vi "DataAcqMaster.vi"(0 "Motion Settings In":T4={"No Motion?"=FALSE, "Motion System"=enum."NI 735x", "Motion Bd ID"=1, "Motion Profile"="SMAC1", "# Axis"=1, "Reverse Z axis?"=TRUE, "SMAC Axis"=0, "scan pair"=enum."y-(x) scan", "RT fps"=6.0, "Steps per mm"=[1000, 1000, 1000, 1000], "Motor Parameters"={"velocity ct/s"=[10000.0, 10000.0, 10000.0, 50000.0], "accel ct/s^2"=[50000.0, 50000.0, 50000.0, 200000.0]}, "One Way Scan"=FALSE, "Reverse One Way Scan"=FALSE, "Global Position (mm)"=[], "Plane"=0, "Distance between\nscan lines (um)"=0.0, "Distance between\nscan planes (um)"=0.0, "number of scan planes"=1, "Total steps in line"=0, "Xtra plane\ndistance  (um)"=100, "Xtra planes "=1, "Add Axis"=FALSE, "overshoot cts"=200, "BKPT Shift"=0, "Scan Start Time (ms)"=0, "ESP VISA"="GPIB::1::INSTR", "3rd Axis"=1, "GL Ref Out"=refnum, "Galil Address"=""} {"3rd Axis" items=["x", "y", "z", "w"]; "Xtra planes" min=1; "Xtra plane\ndistance  (um)" min=0; "Distance between\nscan planes (um)" format="%.2f"; "Distance between\nscan lines (um)" format="%.2f"; "SMAC Axis" items=["None"=0, "Axis 1"=1, "Axis 2"=2, "Axis 3"=3, "Axis 4"=4, "Axis 5"=5, "Axis 6"=6, "Axis 7"=7, "Axis 8"=8, "Vector Space 1"=17, "Vector Space 2"=18, "Vector Space 3"=19, "Vector Space 4"=20]; "Motion Bd ID" min=1 max=32 step=1}, 1 "2-D motor":bool, 2 "Type of scan":T12, 3 "Move motor":bool, 5 "Therapy (T)":bool, 6 "Scan Name":string, 7 "Xmit Ring":i16, 8 "Digitizer Settings":T8={"Digitizer delay (us) "=0.0, "rf points per line"=2048, "lines per plane"=128, "Samp Rate (Hz)"=100000000.0, "Additional dig delay (us)"=0.0, "Voltage Scale"=0.4, "Pre-Looks"=0, "Offset delay (us)"=0.0, "bits A/D"=8, "Avg Num"=1, "DigTimeOut"=5.0, "Rel Dig Delay"=0.0, "Dig Ch"=0, "LeCroyCluster"={"LeCroy Channels"=[TRUE, FALSE, FALSE, FALSE], "LC read pt offset"=0.0, "Sweep Avg"=FALSE}, "Main Digitizer"=enum."NI Digitizer", "Dig Config"=enum."Single channel", "Digitizer ID Cluster"={"Acqiris/Alazar/SP ID"=[], "NI Instr Handles"=[], "LeCroy VISA"="", "GaGe Handle"={"Handle"=0, "Sample size"=0, "Resolution"=0, "Offset"=0, "Channels"=0, "Boards"=0}, "ATS Ref"="ATS9350", "Acqiris Address"=["PCI::INSTR0"], "ADQRef"=refnum, "adq_cu_ptr"=refnum}, "Trigger Settings"={"Trig Source"=1, "Trig Coupling"=0, "Trig Slope"=0, "Level (mV)"=1500.0}, "Bulk Acq"=FALSE, "Bulk Start Indexes"=[], "Data Ref RF"=refnum, "NI ID/Channel"=[], "Total Dig CH"=1, "Xtra Ann Trig delay (us)"=10.0, "Fix Z Delay?"=FALSE, "One Way Transmission?"=FALSE, "Data Ref Log"=refnum} {"Trigger Settings"."Trig Slope" items=["Positive", "Negative"]; "Trigger Settings"."Level (mV)" format="%.2f"; "Trigger Settings"."Trig Coupling" items=["DC 1 MOhm", "AC 1 MOhm", "DC 50 Ohm", "AC 50 Ohm"]; "Trigger Settings"."Trig Source" items=["Chan 1", "External"]; "Rel Dig Delay" format="%.2f"; "DigTimeOut" format="%.2f"; "Avg Num" min=1; "Offset delay (us)" format="%.2f"; "Additional dig delay (us)" format="%.2f"; "Digitizer delay (us)" format="%.2f"}, 10 "lines per plane mod":i32, 12 "Ann Array Params":T1={"Synth Foc?"=FALSE, "Focal Zones"=41, "Switch T/R"=0, "Trans Geometry (mm)"={"Transducer"=0, "Geo Focus"=12.0, "a (radius)"=3.0, "# of rings"=5, "kerf space "=0.1, "Center Freq"=12.0}, "Sub Ap Excite?"=FALSE, "Full Array Scan?"=FALSE, "Xmt/Rcv"={"XMIT"=[TRUE, TRUE, TRUE, TRUE, TRUE], "RCV"=[TRUE, TRUE, TRUE, TRUE, TRUE]}, "PulseSpacing (us)"=0.0, "Xmit Ring"=0, "XMIT CHS"=0, "RCV CHS"=0, "GPU?"=FALSE, "Save TIFF?"=FALSE, "downfactor"=1, "RCV 1CH"=0} {"RCV 1CH" items=["All", "1", "2", "3", "4", "5"]; "Trans Geometry (mm)"."Transducer" items=["6D 12R 40 MHz"=0, "10D 31R 20 MHz"=1, "10D 23R 20 MHz"=2, "6D 23R 40 MHz"=3, "4.5D 10.7R 40 MHz"=4, "9D 23.5R 20 MHz"=5, "9D 25.8R 20MHz"=6, "Enter"=99]; "Switch T/R" min=1 max=5 step=1}, 13 "Reverse ?":bool, 14 "DAQmx Task 2":refnum<k21>, 15 "Full Array Scan?":bool, 16 "start value":dbl, 18 "scan axis":i32) -> (17 "Stop Scan":bool, 21 "Motion error":bool, 22 "Timeout":bool, 26 "error out":errorcluster, 27 "Record Index":i32)   [LabVIEW 2022 SP3]
uses:
  Controls/ScanType2.ctl
  Digitizers/-DigitizerRoutines/DigitizerSettings.ctl
  Digitizers/-DigitizerRoutines/Digitizer.ctl
  Digitizers/-DigitizerRoutines/DigConfig.ctl
  Digitizers/-DigitizerRoutines/DigitizerID.ctl
  C:/Windows/System32/ADQAPI_dotNet_helper.dll
  Windows/System32/ADQAPI_dotNet_helper.dll
  Motion Controllers/NI_controller/-NI_MotionRoutines/MotionParameters.ctl
  Motion Controllers/NI_controller/-NI_MotionRoutines/MotionSys.ctl
  Motion Controllers/-MotionRoutines/ScanAxis.ctl
  Motion Controllers/-MotionRoutines/3rdAxis.ctl
  Annular Array/-AnnularRoutines/AnnularArray.ctl
  Annular Array/-AnnularRoutines/TransGeometry.ctl
  Annular Array/-AnnularRoutines/ArrayGeometry.ctl
  Motion Controllers/Galil/Command Menu.ctl
  Controls/location.ctl
  <vilib>/DAQmx/write.llb/DAQmx Write (Digital Bool 1Line 1Point).vi
  <vilib>/DAQmx/read.llb/DAQmx Read (Analog 2D I16 NChan NSamp).vi
  Motion Controllers/-MotionRoutines/MotionGlobals.vi
  Pulsers/PulserGlobals.vi
  <vilib>/DAQmx/miscellaneous.llb/DAQmx Fill In Error Info.vi
  Switch Modules/SwitchGlobals.vi
  <instrlib>/Acqiris Dx/Acqiris Dx.lvlib
  <vilib>/Motion/FlexMotion/FunctionsVIs/Trajectory.llb/Wait for Move Complete (8 axes).flx
  <resource>/objmgr/daqmx.rc
  <vilib>/Motion/FlexMotion/CustomControls/CustomControls.llb/Mask (8 axes).flx
  <instrlib>/Newport ESP301/Newport ESP301.lvlib
  <instrlib>/LeCroy Wave Series/LeCroy Wave Series.lvlib
  <instrlib>/Agilent 34970/Agilent 34970.lvlib
  <vilib>/Motion/FlexMotion/FunctionsVIs/MotionIO.llb/Set Breakpoint Output MOMO (8 axes).flx
  <vilib>/Motion/FlexMotion/FunctionsVIs/MotionIO.llb/Set Inhibit MOMO (8 axes).flx
panel:
  out "TEMP Log 2":bool
  # "1-D and 2-D B scan settings"
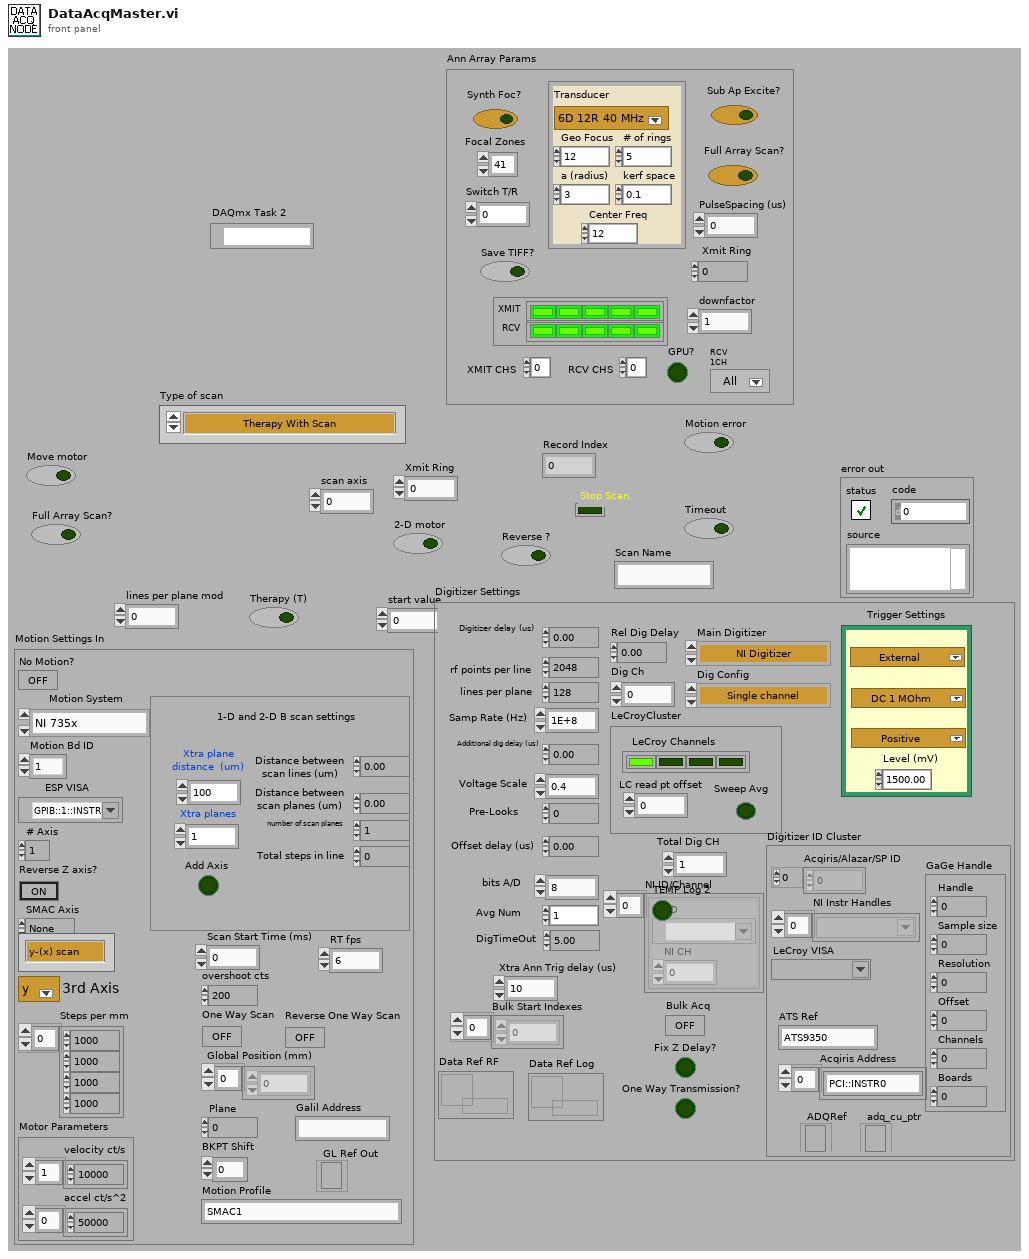
[diagram p1: front panel]
types:
  T1 = typedef "AnnularArray.ctl" = cluster{"Synth Foc?":bool, "Focal Zones":i16, "Switch T/R":i16, "Trans Geometry (mm)":T2, "Sub Ap Excite?":bool, "Full Array Scan?":bool, "Xmt/Rcv":cluster{"XMIT":bool[], "RCV":bool[]}, "PulseSpacing (us)":sgl, "Xmit Ring":i32, "XMIT CHS":u8, "RCV CHS":u8, "GPU?":bool, "Save TIFF?":bool, "downfactor":i32, "RCV 1CH":u16}
  T2 = typedef "TransGeometry.ctl" = cluster{"Transducer":T3, "Geo Focus":dbl, "a (radius)":dbl, "# of rings":i32, "kerf space ":dbl, "Center Freq":dbl}
  T3 = typedef "ArrayGeometry.ctl" = u16
  T4 = typedef "MotionParameters.ctl" = cluster{"No Motion?":bool, "Motion System":T5, "Motion Bd ID":u8, "Motion Profile":string, "# Axis":i8, "Reverse Z axis?":bool, "SMAC Axis":u16, "scan pair":T6, "RT fps":sgl, "Steps per mm":i32[], "Motor Parameters":cluster{"velocity ct/s":dbl[], "accel ct/s^2":dbl[]}, "One Way Scan":bool, "Reverse One Way Scan":bool, "Global Position (mm)":dbl[], "Plane":i32, "Distance between\nscan lines (um)":sgl, "Distance between\nscan planes (um)":sgl, "number of scan planes":i32, "Total steps in line":i32, "Xtra plane\ndistance  (um)":i32, "Xtra planes ":i32, "Add Axis":bool, "overshoot cts":i32, "BKPT Shift":i32, "Scan Start Time (ms)":u32, "ESP VISA":refnum<visa-resource-name>, "3rd Axis":T7, "GL Ref Out":refnum<k7>, "Galil Address":string}
  T5 = typedef "MotionSys.ctl" = enum16{"MM3000", "NI 735x", "Newport ESP", "No Motion Card", "Galil"}
  T6 = typedef "ScanAxis.ctl" = enum16{"y-(x) scan", "x-(y) scan", "z-(x) scan", "z-(y) scan", "y-(z) scan", "x-(z) scan", "w-(x) scan", "w-(y) scan", "w-(z) scan", "x-(w) scan", "y-(w) scan", "z-(w) scan"}
  T7 = typedef "3rdAxis.ctl" = u16
  T8 = typedef "DigitizerSettings.ctl" = cluster{"Digitizer delay (us) ":dbl, "rf points per line":i32, "lines per plane":i32, "Samp Rate (Hz)":dbl, "Additional dig delay (us)":dbl, "Voltage Scale":dbl, "Pre-Looks":i32, "Offset delay (us)":dbl, "bits A/D":i8, "Avg Num":i32, "DigTimeOut":sgl, "Rel Dig Delay":sgl, "Dig Ch":i32, "LeCroyCluster":cluster{"LeCroy Channels":bool[], "LC read pt offset":dbl, "Sweep Avg":bool}, "Main Digitizer":T9, "Dig Config":T10, "Digitizer ID Cluster":T11, "Trigger Settings":cluster{"Trig Source":u16, "Trig Coupling":u16, "Trig Slope":u16, "Level (mV)":dbl}, "Bulk Acq":bool, "Bulk Start Indexes":i32[], "Data Ref RF":refnum<data-value>, "NI ID/Channel":cluster{"NI ID":refnum<k15>, "NI CH":i32}[], "Total Dig CH":i32, "Xtra Ann Trig delay (us)":dbl, "Fix Z Delay?":bool, "One Way Transmission?":bool, "Data Ref Log":refnum<data-value>}
  T9 = typedef "Digitizer.ctl" = enum16{"Acqiris Digitizer", "NI Digitizer", "LeCroy", "GaGe", "AlazarTech", "No Digitizer", "Teledyne"}
  T10 = typedef "DigConfig.ctl" = enum16{"Single channel", "2 Chans w/ 2 Acqiris", "2 Chans w/ 1 Acqiris", "5-CH Pulser New", "5-CH pulser w/ ann array", "5-pass style ann array", "Empty"}
  T11 = typedef "DigitizerID.ctl" = cluster{"Acqiris/Alazar/SP ID":u32[], "NI Instr Handles":refnum<k15>[], "LeCroy VISA":refnum<visa-resource-name>, "GaGe Handle":cluster{"Handle":u32, "Sample size":u32, "Resolution":i32, "Offset":i32, "Channels":u32, "Boards":u32}, "ATS Ref":string, "Acqiris Address":string[], "ADQRef":refnum<k24>, "adq_cu_ptr":refnum<k24>}
  T12 = typedef "ScanType2.ctl" = enum16{"Therapy With Scan", "M scan", "M Scan With Therapy Burst", "1-D B Scan", "1-D B Scan With Therapy Burst", "2-D B Scan", "2-D B Scan With Therapy Burst", "Rotational Scan", "1-D B-Scan PRF", "2-D B-Scan PRF", "Real-Time Scan", "Contrast Agents", "1-D w/ Real-Time Set Up", "Dual Transducer", "Acoustic Microscopy", "Hydrophone Scanning"}
  T13 = typedef "EKG_Mode.ctl" = u16
  T14 = typedef "Mask (8 axes).flx" = cluster{"1":bool, "2":bool, "3":bool, "4":bool, "5":bool, "6":bool, "7":bool, "8":bool}
  T15 = typedef "Command Menu.ctl" = enum16{"CommandPassThrough", "Abort Motion", "Define Pos", "Velocity", "Acceleration", "Deceleration", "Position Rel", "Postion Abs", "Begin Move", "After Move", "Home", "KI", "KD", "KP", "IL", "Config I/O", "Set Bit", "Clear Bit", "Motor Off", "Moto On", "Status", "Execute", "Halt Execute", "HX Status", "Tell Velocity", "Check Motion", "BreakPoint", "Tell Position", "Current Code Line", "Tell Switches", "OC Force On", "OC Off", "Pos Soft Limit", "Rev Soft Limit"}
  T16 = typedef "location.ctl" = enum16{"Automatic", "WCM Main", "Hawaii", "Columbia MM3000", "Columbia  NI System", "NYU", "RRI 2", "UHI Allen", "CUMC RT", "Chiba", "Stony Brook", "WCM Microscopy", "WCM Aeoretch", "WCM Optics Lab", "WCM Main 2Axis", "WCM Rotation", "WCM SAM SMAC", "SERI GP"}
  T17 = cluster{dbl, "Clock mode":enum16{"Internal", "External", "Reference"}, "RingText.Text":string, i32, i32, "time out (ms)":dbl, dbl, dbl}
  T18 = enum16{"big-endian, network order", "native, host order", "little-endian"}
  T19 = enum16{"open", "replace", "create", "open or create", "replace or create", "replace or create with confirmation"}
  T20 = cluster{"Therapy frequency (MHz)":dbl, "Therapy amplitude (mV)":dbl, "time therapy on (s)":dbl, "Therapy Delay (ms) ":dbl, "Time (s)":dbl}
  T21 = enum32{"unused", "DC, 1 MOhm", "AC, 1 MOhm", "DC, 50 Ohm", "AC 50 Ohm"}
  T22 = cluster{"Handle":u32, "Sample size":u32, "Resolution":i32, "Offset":i32, "Channels":u32, "Boards":u32}
  T23 = cluster{"Voltage Scale":dbl, "Voltage Scale":dbl, "Crate Coupling":u16}
  T24 = cluster{"data value reference":refnum<data-value>, "bytes to transfer":u32, "rf pts actual":u32}
  T25 = cluster{"Port A bit-0 at logic level":bool, "Port A bit-1 at logic level":bool, "Port A bit-2 at logic level ":bool, "Port A bit-3 at logic level":bool, "Port A bit-4 at logic level":bool, "Port A bit-5 at logic level ":bool, "Port A bit-6 at logic level ":bool, "Port A bit-7 at logic level ":bool, "Port B bit-0 at logic level":bool, "Port B bit-1 at logic level":bool, "Port B bit-2 at logic level ":bool, "Port B bit-3 at logic level":bool, "Port B bit-4 at logic level":bool, "Port B bit-5 at logic level ":bool, "Port B bit-6 at logic level ":bool, "Port B bit-7 at logic level ":bool}
  T26 = typedef "SwitchOption.ctl" = enum16{"Cytex", "Pickering", "NI Switch", "No Switch", "Riverside USB"}
  T27 = typedef "Bd Id Out" = u8
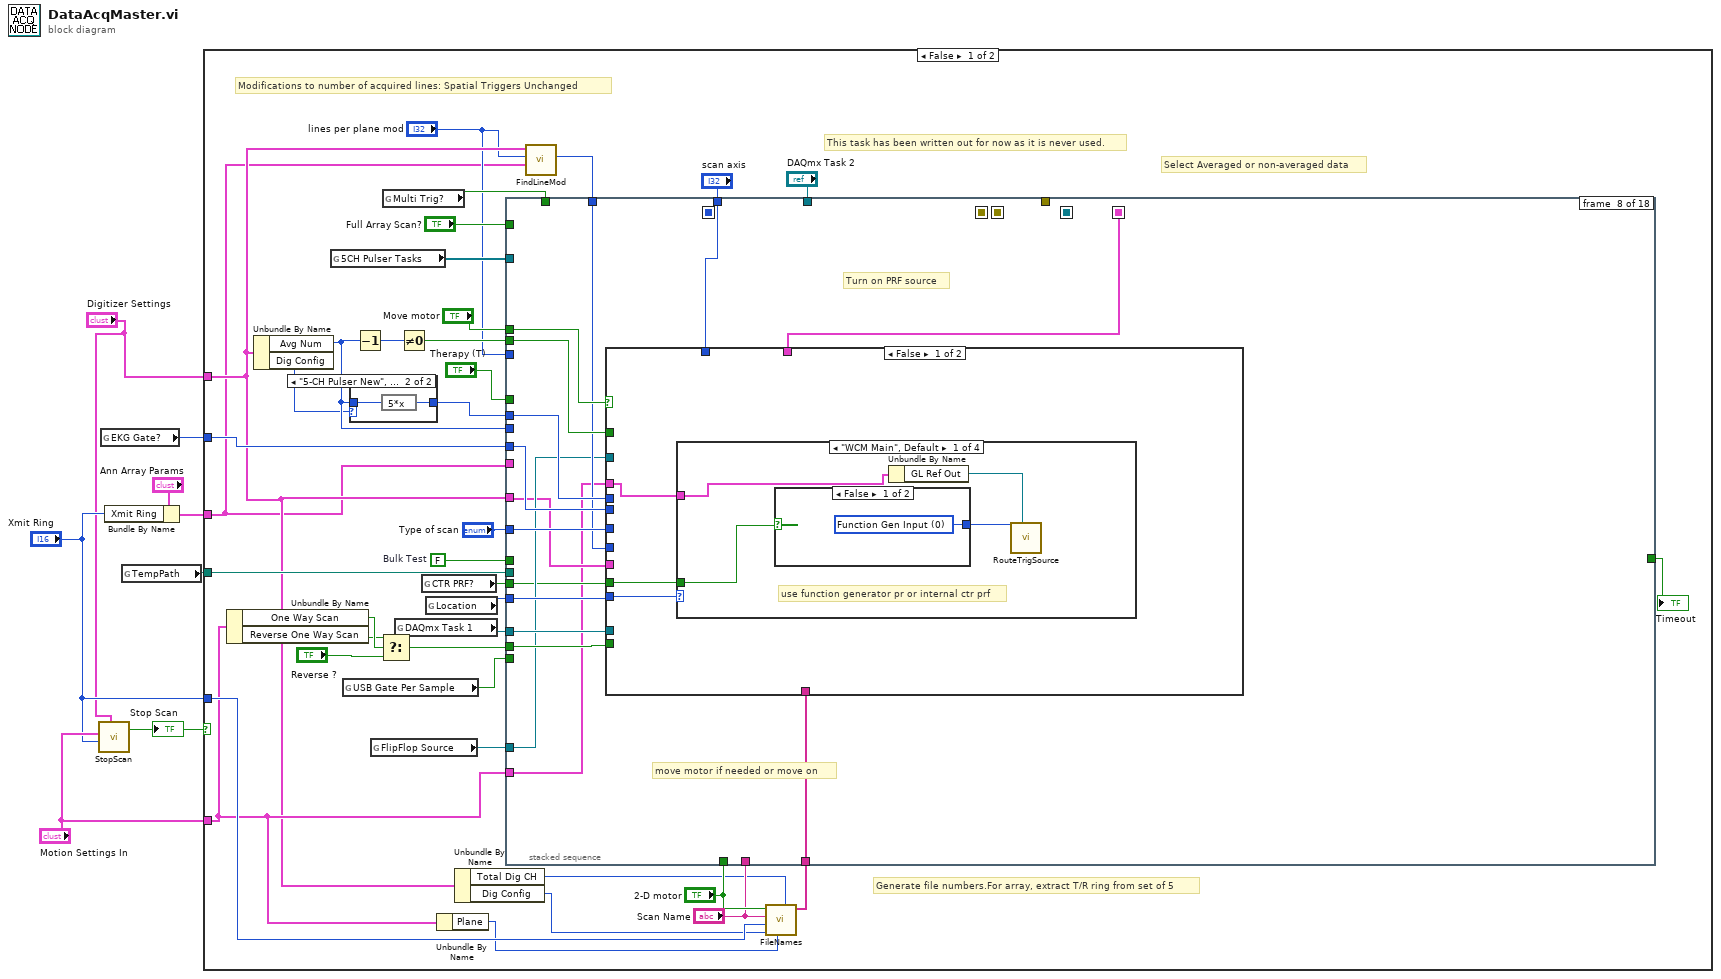
[diagram p0: block diagram]
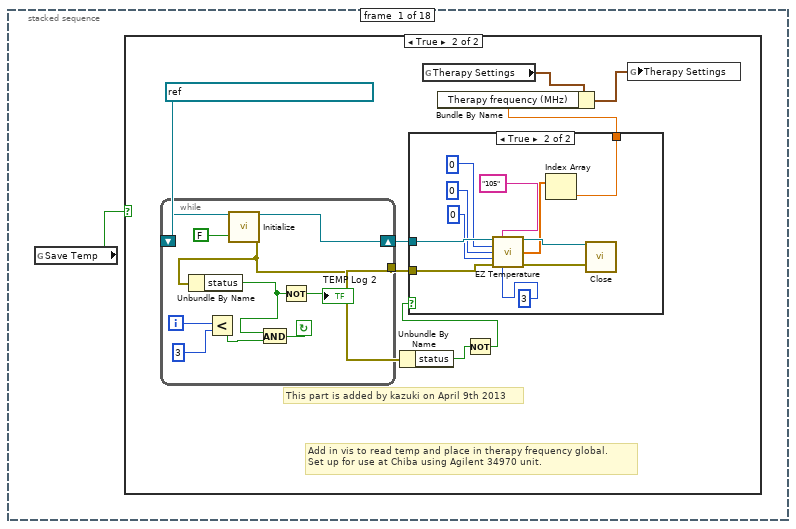
[diagram p3: hidden frame]
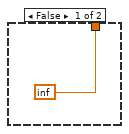
[diagram p5: hidden frame]
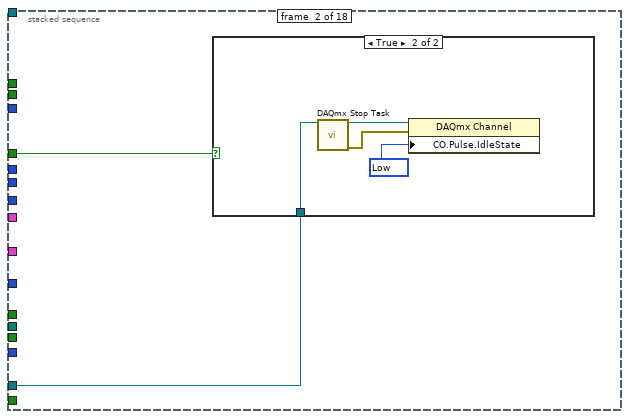
[diagram p6: hidden frame]
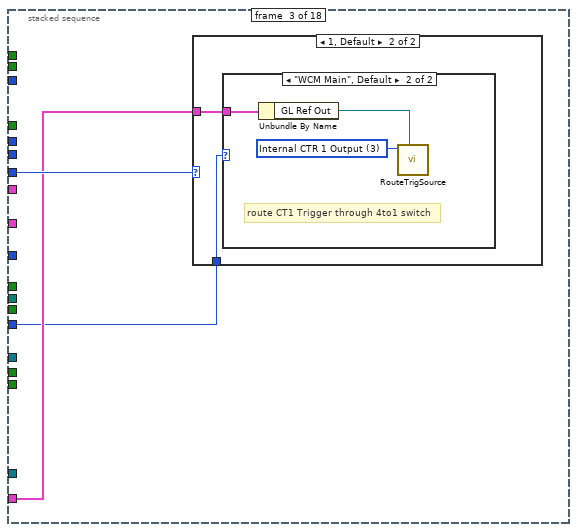
[diagram p8: hidden frame]
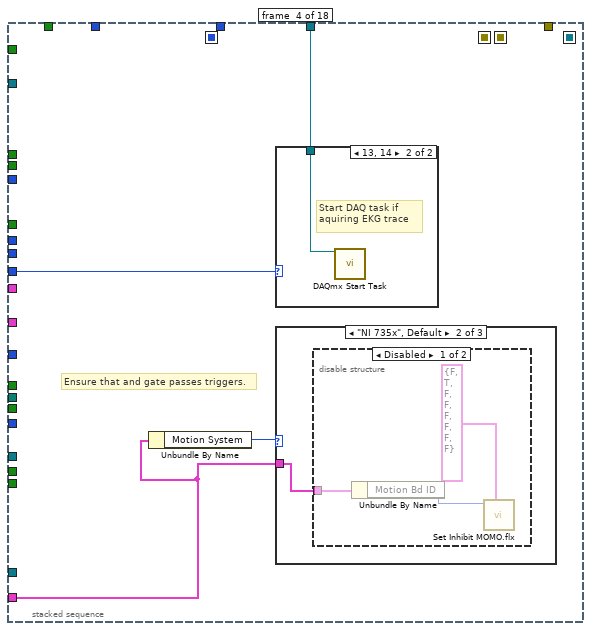
[diagram p11: hidden frame]
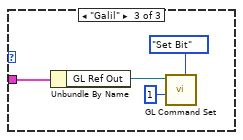
[diagram p14: hidden frame]
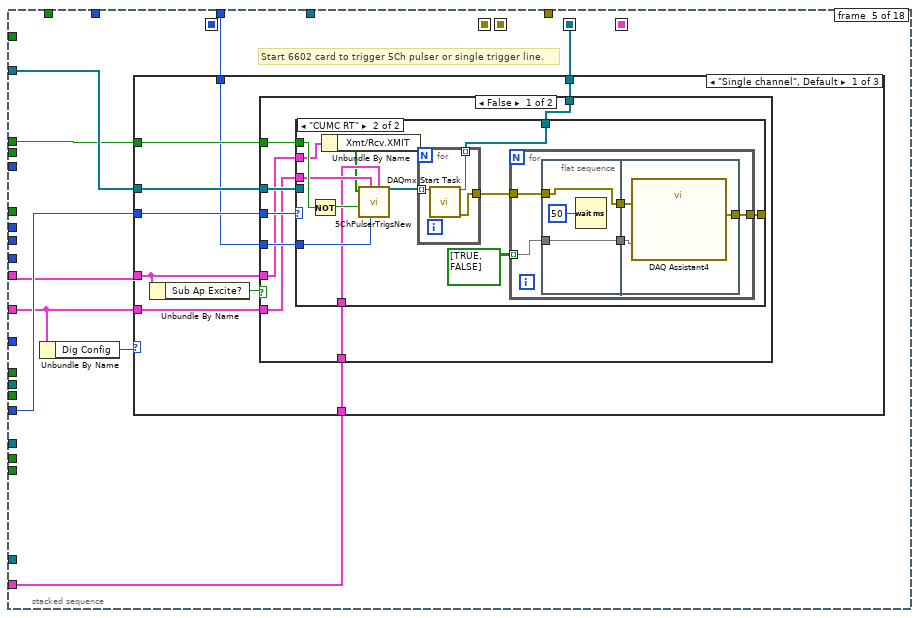
[diagram p16: hidden frame]
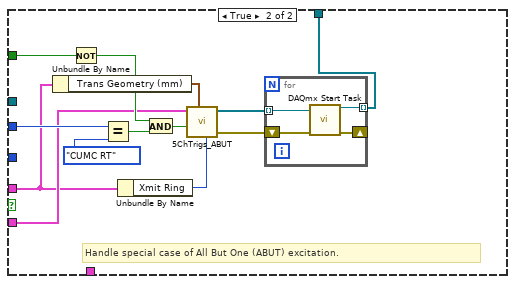
[diagram p18: hidden frame]
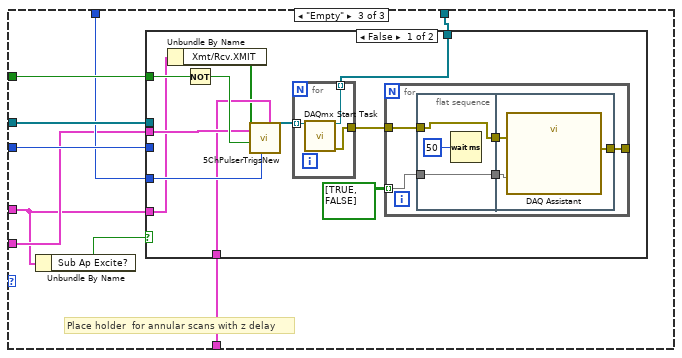
[diagram p20: hidden frame]
diagram:
  n1 = call "StopScan.vi"("Motion Settings In"="Motion Settings In", "Ring"="Xmit Ring", "Digitizer Settings"="Digitizer Settings") -> ("Stop Now? Dup"=w8:bool)  [unwired: 3 in]
  "Stop Scan" <- w8
  n2 = global read "MotionGlobals.vi" "EKG Gate?"() -> (w7:T13)
  n3 = Bundle By Name(cluster="Ann Array Params", "Xmit Ring"="Xmit Ring") -> (w2:T1)
  n4 = global read "MotionGlobals.vi" "TempPath"() -> (w6:path)
  n5 = case shown="False" w8 {
    tunnel: "Xmit Ring" -> [w16 _]
    tunnel: w7 -> [w46 _]
    tunnel: w6 -> [w28 _]
    tunnel: "Digitizer Settings" -> [w11 _]
    tunnel: "Motion Settings In" -> [w14 _]
    tunnel: w2 -> [w9 _]
    frame False {
      w32 = FALSE  # Bulk Test
      # "This task has been written out for now as it is never used."
      # "Modifications to number of acquired lines: Spatial Triggers Unchanged"
      # "Generate file numbers.For array, extract T/R ring from set of 5"
      # "Select Averaged or non-averaged data"
      n6 = Unbundle By Name(w14) -> ("One Way Scan"=w20:bool, "Reverse One Way Scan"=w18:bool)
      n7 = Unbundle By Name(w11) -> ("Avg Num"=w22:i32, "Dig Config"=w21:T10)
      n8 = global read "MotionGlobals.vi" "5CH Pulser Tasks"() -> (w29:refnum<k21>[])
      n9 = global read "MotionGlobals.vi" "USB Gate Per Sample"() -> (w19:bool)
      n10 = case shown="\"5-CH Pulser New\", \"5-CH pulser w/ ann array\"" w21 {
        tunnel: [w47 w49] -> w27
        tunnel: w22 -> [w47 w48]
        frame "Single channel", Default {
        }
        frame "5-CH Pulser New", "5-CH pulser w/ ann array" {
          n11 = expression code="5*x"(w48) -> (w49:i32)
        }
      }
      n12 = Decrement(x=w22) -> (x-1=w40:i32)
      n13 = global read "MotionGlobals.vi" "FlipFlop Source"() -> (w26:refnum<k21>)
      n14 = Select(t=w18, s=w20, f="Reverse ?") -> (s? t:f=w35:bool)
      n15 = global read "MotionGlobals.vi" "Multi Trig?"() -> (w23:bool)
      n16 = global read "MotionGlobals.vi" "DAQmx Task 1"() -> (w37:refnum<k21>)
      n17 = Not Equal To 0?(x=w40) -> (x != 0?=w41:bool)
      n18 = global read "MotionGlobals.vi" "CTR PRF?"() -> (w25:bool)
      n19 = global read "MotionGlobals.vi" "Location"() -> (w39:T16)
      n20 = Unbundle By Name(w14) -> ("Plane"=w13:i32)
      n21 = Unbundle By Name(w11) -> ("Total Dig CH"=w17:i32, "Dig Config"=w15:T10)
      n22 = call "FindLineMod.vi"("Ann Array Params"=w9, "lines per plane in"="lines per plane mod", "Digitizer Settings"=w11) -> ("lines per plane mod out"=w24:i32)  [unwired: 8 in]
      n23 = call "FileNames.vi"("# Elements"=w17, "Plane"=w13, "Dig Config"=w15, "Xmit Ring"=w16, "Scan Name"="Scan Name", "2-D motor"="2-D motor") -> ("All files"=w34:string[])  [unwired: 3 in, 2 out]
      n24 = stacked-sequence {
        seq-local: [_ _ _ _ _ w245 _ _ _ _ _ _ _ _ _ _ _ _] -> [_ _ _ _ _ _ _ _ w566 _ _ _ _ _ _ _ _ _]
        seq-local: [_ _ _ _ _ _ _ _ w559 _ _ _ _ _ _ _ _ _] -> [_ _ _ _ _ _ _ _ _ w635 w682 _ _ _ _ _ _ _]
        seq-local: [_ _ _ _ _ w241 _ _ _ _ _ _ _ _ _ _ _ _] -> [_ _ _ _ _ _ _ _ w563 w633 w680 _ _ _ _ _ _ _]
        seq-local: [_ _ _ _ w113 _ _ _ _ _ _ _ _ _ _ _ _ _] -> [_ _ _ _ _ _ _ _ _ _ _ _ _ w803 _ _ _ _]
        seq-local: [_ _ _ _ _ w236 _ _ _ _ _ _ _ _ _ _ _ _] -> [_ _ _ _ _ _ _ w464 _ _ w674 _ _ _ _ _ _ w1004]
        tunnel: "Therapy (T)" -> [_ w81 _ _ _ _ w453 _ _ _ _ _ w779 _ _ _ _ _]
        tunnel: "Move motor" -> [_ _ _ _ w114 _ w450 w477 _ _ _ _ w776 _ _ w872 _ _]
        tunnel: "scan axis" -> [_ _ _ _ w112 _ _ w475 _ _ w677 _ _ _ _ w868 w931 _]
        tunnel: w35 -> [_ _ _ _ _ _ _ w476 _ w634 w681 _ _ _ _ w870 _ _]
        tunnel: [_ _ _ _ _ _ _ _ w565 _ _ _ _ _ _ _ _ _] -> w45
        tunnel: "Type of scan" -> [_ _ _ _ _ _ w447 w472 _ w625 w670 _ w774 _ _ _ w926 _]
        tunnel: w41 -> [_ _ _ _ _ w243 _ w474 _ _ _ _ _ _ _ _ _ _]
        tunnel: w27 -> [_ _ _ _ _ w244 _ w473 w564 _ _ _ _ _ _ _ _ _]
        tunnel: w39 -> [_ _ w87 _ w115 _ w444 w471 _ _ _ _ w770 w804 _ w871 _ _]
        tunnel: w37 -> [_ w82 _ _ _ _ w455 w467 _ _ _ _ w783 _ _ _ _ _]
        tunnel: w46 -> [_ _ w89 w98 _ _ _ w470 _ w632 w679 _ w782 _ w825 w869 w928 _]
        tunnel: w24 -> [_ _ _ _ _ w242 _ w469 w562 _ _ _ _ _ _ _ _ _]
        tunnel: w23 -> [_ _ _ _ _ _ w454 _ _ _ _ _ w771 _ _ _ _ _]
        tunnel: w34 -> [_ _ _ _ _ _ _ w468 _ _ w678 _ _ _ w824 _ _ _]
        tunnel: "Full Array Scan?" -> [_ _ _ _ _ _ _ _ _ _ _ w754 _ _ _ _ _ _]
        tunnel: "DAQmx Task 2" -> [_ _ _ w97 _ _ _ _ _ _ _ _ _ _ w823 _ _ _]
        tunnel: w32 -> [_ _ _ _ _ _ _ _ _ w631 w676 _ _ _ _ _ _ _]
        tunnel: "2-D motor" -> [_ _ _ _ _ _ _ _ _ w630 _ _ _ _ _ _ _ _]
        tunnel: "Scan Name" -> [_ _ _ _ _ _ _ _ _ w629 _ _ _ _ _ _ _ _]
        tunnel: w29 -> [_ _ _ _ w116 _ _ _ _ _ _ _ _ _ _ _ _ _]
        tunnel: w28 -> [_ _ _ _ _ _ _ _ _ _ _ _ _ _ w822 _ _ _]
        tunnel: w22 -> [_ _ _ _ _ w237 _ _ _ _ w675 _ _ _ _ _ _ _]
        tunnel: w26 -> [_ _ _ _ _ _ _ w466 _ _ _ _ _ _ _ _ _ w1005]
        tunnel: w25 -> [_ _ _ _ _ _ w451 w465 _ _ _ _ w778 _ _ _ _ _]
        tunnel: w11 -> [_ _ _ _ w109 w230 _ w463 w561 w628 w673 w750 _ w801 w821 _ _ w1000]
        tunnel: w14 -> [_ _ w88 w96 w111 w231 _ w462 _ w627 w672 _ w772 _ _ w867 w924 w1003]
        tunnel: w19 -> [_ _ _ _ _ _ w448 _ w560 _ _ _ _ _ _ _ _ _]
        tunnel: w9 -> [_ _ _ _ w110 w235 _ _ _ w626 w671 w752 _ w802 w820 _ _ _]
        tunnel: [_ _ _ _ _ _ _ _ w559 _ _ _ _ _ _ _ _ _] -> _
        tunnel: "lines per plane mod" -> [_ _ _ _ _ _ _ _ _ _ _ _ _ _ w819 _ _ _]
        frame #0 {
          n25 = global read "MotionGlobals.vi" "Save Temp"() -> (w50:bool)
          n26 = case shown="True" w50 {
            frame False {
            }
            frame True {
              # "This part is added by kazuki on April 9th 2013"
              # "Add in vis to read temp and place in therapy frequency global.\nSet up for use at Chiba using Agilent 34970 unit."
              n27 = while {
                tunnel: [w77] -> w56
                shift-right: [w79] -> w58
                shift-left: refnum<visa-resource-name> "TCPIP0::192.168.1.170::inst0::INSTR" ("VISA Resource Name") -> [w78]
                i -> [w74]
                stop <- w76 continue-if-true
                n28 = Less?(x=w74, y=3) -> (x < y?=w75:bool)
                n29 = call <instrlib>:"Initialize.vi"("VISA Resource Name"=w78, "Reset (T: Reset)"=FALSE) -> ("VISA Resource Name Out"=w79:refnum<visa-resource-name>, "error out"=w77:errorcluster)  [unwired: 12 in]
                n30 = Unbundle By Name(w77) -> ("status"=w71:bool)
                n31 = And(x=w71, y=w75) -> (x .and. y?=w76:bool)
                n32 = Not(x=w71) -> (.not. x?=→"TEMP Log 2":bool)
              }
              n33 = Unbundle By Name(w56) -> ("status"=w55:bool)
              n34 = global read "PulserGlobals.vi" "Therapy Settings"() -> (w53:T20)
              n35 = Not(x=w55) -> (.not. x?=w54:bool)
              n36 = case shown="True" w54 {
                tunnel: [inf w67] -> w52
                tunnel: w58 -> [_ w65]
                tunnel: w56 -> [_ w60]
                frame False {
                }
                frame True {
                  n37 = call <instrlib>:"EZ Temperature.vi"("VISA Resource Name"=w65, "Scan List (empty)"="105", "Thermocouple Type (8:Def-Last)"=0, "Thermistor Type (3:Def-Last)"=0, "RTD Type (2:Default-Last)"=0, "error in (no error)"=w60, "Transducer Type (4:Def-Last)"=3) -> ("VISA Resource Name Out"=w69:refnum<visa-resource-name>, "Output Array"=w68:dbl[], "error out"=w70:errorcluster)  [unwired: 6 in]
                  n38 = Index Array(array=w68) -> (element=w67:dbl)  [unwired: 1 in]
                  n39 = call <instrlib>:"Close.vi"("VISA Resource Name"=w69, "error in (no error)"=w70) -> ()  [unwired: 13 in, 1 out]
                }
              }
              n40 = Bundle By Name(cluster=w53, "Therapy frequency (MHz)"=w52) -> (w51:T20)
              n41 = global write "PulserGlobals.vi" "Therapy Settings"(w51) -> ()
            }
          }
        }
        frame #1 {
          n42 = case shown="True" w81 {
            tunnel: w82 -> [_ w86]
            frame False {
            }
            frame True {
              w83 = 10214 items=["High"=10192, "Low"=10214] ("CO.Pulse.IdleState")
              n43 = call <vilib>:"DAQmx Stop Task.vi"("task/channels in"=w86) -> ("task out"=w85:refnum<k21>, "error out"=w84:errorcluster)  [unwired: 1 in, 12 out]
              n44 = property class="DAQmx Channel"(reference=w85, error in=w84, "CO.Pulse.IdleState"=w83) -> ()  [unwired: 2 out]
            }
          }
        }
        frame #2 {
          n45 = case shown="1, Default" w89 {
            tunnel: w88 -> [_ w91]
            tunnel: w87 -> [_ w90]
            frame 0 {
            }
            frame 1, Default {
              n46 = case shown="\"WCM Main\", Default" w90 {
                tunnel: w91 -> [_ w93]
                frame "SERI GP" {
                }
                frame "WCM Main", Default {
                  w94 = u16 3 items=["Function Gen Input", "Motion Trig", "Internal RT Motion Trig", "Internal CTR 1 Output"] ("Trig Source")
                  # "route CT1 Trigger through 4to1 switch"
                  n47 = Unbundle By Name(w93) -> ("GL Ref Out"=w92:refnum<k7>)
                  n48 = call "RouteTrigSource.vi"("Galil.IGalil"=w92, "Trig Source"=w94) -> ()  [unwired: 9 in, 1 out]
                }
              }
            }
          }
        }
        frame #3 {
          # "Ensure that and gate passes triggers."
          n49 = Unbundle By Name(w96) -> ("Motion System"=w95:T5)
          n50 = case shown="13, 14" w98 {
            tunnel: w97 -> [_ w107]
            frame 0, Default {
            }
            frame 13, 14 {
              # "Start DAQ task if aquiring EKG trace"
              n51 = call <vilib>:"DAQmx Start Task.vi"("task/channels in"=w107) -> ()  [unwired: 1 in, 14 out]
            }
          }
          n52 = case shown="\"NI 735x\", Default" w95 {
            tunnel: w96 -> [_ w99 w104]
            frame "MM3000", "Newport ESP", "No Motion Card" {
            }
            frame "NI 735x", Default {
              n53 = disable-structure shown="Disabled" {
                disable-tunnel: w99 -> [w101 _]
                frame Disabled {
                  n54 = Unbundle By Name(w101) -> ("Motion Bd ID"=w100:u8)
                  n55 = call-poly <vilib>:"Set Inhibit MOMO.flx"("Must On (False)"=T14 {"1"=FALSE, "2"=TRUE, "3"=FALSE, "4"=FALSE, "5"=FALSE, "6"=FALSE, "7"=FALSE, "8"=FALSE}, "Board ID"=w100) -> ()  [unwired: 2 in, 6 out]
                }
                frame Enabled {
                }
              }
            }
            frame "Galil" {
              n56 = Unbundle By Name(w104) -> ("GL Ref Out"=w106:refnum<k7>)
              n57 = call "GL Command Set.vi"("Command"=Command_Menu."Set Bit", "Value"=1, "Galil.IGalil"=w106) -> ()  [unwired: 4 in, 5 out]
            }
          }
        }
        frame #4 {
          # "Start 6602 card to trigger 5Ch pulser or single trigger line."
          n58 = Unbundle By Name(w109) -> ("Dig Config"=w108:T10)
          n59 = case shown="\"Single channel\", Default" w108 {
            tunnel: w116 -> [w124 w177 w185]
            tunnel: w115 -> [w125 _ w186]
            tunnel: w114 -> [w123 _ w184]
            tunnel: [w122 w177 w183] -> w113
            tunnel: w112 -> [w121 _ w182]
            tunnel: w109 -> [w118 _ w181]
            tunnel: w111 -> [w120 _ w180]
            tunnel: w110 -> [w117 _ w178]
            frame "Single channel", Default {
              n60 = Unbundle By Name(w117) -> ("Sub Ap Excite?"=w119:bool)
              n61 = case shown="False" w119 {
                tunnel: w125 -> [w133 w168]
                tunnel: w124 -> [w132 _]
                tunnel: w123 -> [w130 w171]
                tunnel: [w129 w165] -> w122
                tunnel: w121 -> [w131 _]
                tunnel: w118 -> [w128 w164]
                tunnel: w120 -> [w127 _]
                tunnel: w117 -> [w126 w160]
                frame False {
                  n62 = case shown="\"CUMC RT\"" w133 {
                    tunnel: w132 -> [_ _]
                    tunnel: w131 -> [_ w144]
                    tunnel: w130 -> [_ w143]
                    tunnel: [_ w141] -> w129
                    tunnel: [_ w138] -> _
                    tunnel: w128 -> [_ w137]
                    tunnel: w127 -> [_ w136]
                    tunnel: w126 -> [_ w134]
                    frame "WCM Main", Default {
                    }
                    frame "CUMC RT" {
                      n63 = Not(x=w143) -> (.not. x?=w145:bool)
                      n64 = Unbundle By Name(w134) -> ("Xmt/Rcv.XMIT"=w135:bool[])
                      n65 = call "5ChPulserTrigsNew.vi"("Motion Settings"=w136, "Digitizer Settings"=w137, "XMIT"=w135, "Axis"=w144, "M-mode?"=w145) -> ("5CH Pulser Tasks"=w142:refnum<k21>[])  [unwired: 4 in, 1 out]
                      n66 = for {
                        tunnel: w142 -> [w159] mode=indexing
                        tunnel: [w158] -> w141 mode=indexing
                        tunnel: [w157] -> w139
                        n67 = call <vilib>:"DAQmx Start Task.vi"("task/channels in"=w159) -> ("task out"=w158:refnum<k21>, "error out"=w157:errorcluster)  [unwired: 1 in, 12 out]
                      }
                      n68 = for {
                        tunnel: bool[][] [[TRUE], [FALSE]] ("data") -> [w149] mode=indexing
                        tunnel: [w148] -> w138
                        tunnel: w139 -> [w146]
                        n69 = flat-sequence {
                          tunnel: w149 -> [w153]
                          tunnel: [w153] -> w150
                          tunnel: [w151] -> w147
                          tunnel: w146 -> [w151]
                          tunnel: w150 -> [w156]
                          tunnel: [w155] -> w148
                          tunnel: w147 -> [w154]
                          frame #0 {
                            n70 = Wait (ms)(milliseconds to wait=u32 50) -> ()  [unwired: 1 out]
                          }
                          frame #1 {
                            n71 = call "DAQ Assistant4"("data"=w156, "error in"=w154) -> ("error out"=w155:errorcluster)  [unwired: 16 in, 1 out]
                          }
                        }
                      }
                    }
                  }
                }
                frame True {
                  # "Handle special case of All But One (ABUT) excitation."
                  n72 = Unbundle By Name(w160) -> ("Trans Geometry (mm)"=w162:T2)
                  n73 = Not(x=w171) -> (.not. x?=w170:bool)
                  n74 = Equal?(x=w168, y=location."CUMC RT" ("Location")) -> (x = y?=w169:bool)
                  n75 = Unbundle By Name(w160) -> ("Xmit Ring"=w161:i32)
                  n76 = And(x=w170, y=w169) -> (x .and. y?=w167:bool)
                  n77 = call "5ChTrigs_ABUT.vi"("xmit ring"=w161, "Trans Geometry (mm)"=w162, "Digitizer Settings"=w164, "M-mode?"=w167) -> ("5CH Pulser Tasks"=w166:refnum<k21>[], "error out"=w172:errorcluster)  [unwired: 5 in]
                  n78 = for {
                    tunnel: w166 -> [w176] mode=indexing
                    shift-right: [w174] -> _
                    shift-left: w172 -> [w175]
                    tunnel: [w173] -> w165 mode=indexing
                    n79 = call <vilib>:"DAQmx Start Task.vi"("task/channels in"=w176, "error in"=w175) -> ("task out"=w173:refnum<k21>, "error out"=w174:errorcluster)  [unwired: 12 in]
                  }
                }
              }
            }
            frame "5-CH pulser w/ ann array" {
            }
            frame "Empty" {
              # "Place holder  for annular scans with z delay"
              n80 = Unbundle By Name(w178) -> ("Sub Ap Excite?"=w179:bool)
              n81 = case shown="False" w179 {
                tunnel: w186 -> [_ w220]
                tunnel: w185 -> [_ _]
                tunnel: w184 -> [w196 w223]
                tunnel: [w195 w217] -> w183
                tunnel: w182 -> [w197 _]
                tunnel: w181 -> [w190 w216]
                tunnel: w180 -> [w189 _]
                tunnel: w178 -> [w187 w212]
                frame False {
                  n82 = Unbundle By Name(w187) -> ("Xmt/Rcv.XMIT"=w188:bool[])
                  n83 = Not(x=w196) -> (.not. x?=w194:bool)
                  n84 = call "5ChPulserTrigsNew.vi"("Motion Settings"=w189, "Digitizer Settings"=w190, "XMIT"=w188, "Axis"=w197, "M-mode?"=w194) -> ("5CH Pulser Tasks"=w193:refnum<k21>[])  [unwired: 4 in, 1 out]
                  n85 = for {
                    tunnel: w193 -> [w211] mode=indexing
                    tunnel: [w210] -> w195 mode=indexing
                    tunnel: [w209] -> w191
                    n86 = call <vilib>:"DAQmx Start Task.vi"("task/channels in"=w211) -> ("task out"=w210:refnum<k21>, "error out"=w209:errorcluster)  [unwired: 1 in, 12 out]
                  }
                  n87 = for {
                    tunnel: bool[][] [[TRUE], [FALSE]] ("data") -> [w201] mode=indexing
                    tunnel: [w200] -> _
                    tunnel: w191 -> [w198]
                    n88 = flat-sequence {
                      tunnel: w201 -> [w205]
                      tunnel: [w205] -> w202
                      tunnel: [w203] -> w199
                      tunnel: w198 -> [w203]
                      tunnel: w202 -> [w208]
                      tunnel: [w207] -> w200
                      tunnel: w199 -> [w206]
                      frame #0 {
                        n89 = Wait (ms)(milliseconds to wait=u32 50) -> ()  [unwired: 1 out]
                      }
                      frame #1 {
                        n90 = call "DAQ Assistant"("data"=w208, "error in"=w206) -> ("error out"=w207:errorcluster)  [unwired: 16 in, 1 out]
                      }
                    }
                  }
                }
                frame True {
                  # "Handle special case of All But One (ABUT) excitation."
                  n91 = Not(x=w223) -> (.not. x?=w222:bool)
                  n92 = Unbundle By Name(w212) -> ("Xmit Ring"=w213:i32)
                  n93 = Equal?(x=w220, y=location."CUMC RT" ("Location")) -> (x = y?=w221:bool)
                  n94 = Unbundle By Name(w212) -> ("Trans Geometry (mm)"=w214:T2)
                  n95 = And(x=w222, y=w221) -> (x .and. y?=w219:bool)
                  n96 = call "5ChTrigs_ABUT.vi"("xmit ring"=w213, "Trans Geometry (mm)"=w214, "Digitizer Settings"=w216, "M-mode?"=w219) -> ("5CH Pulser Tasks"=w218:refnum<k21>[], "error out"=w224:errorcluster)  [unwired: 5 in]
                  n97 = for {
                    tunnel: w218 -> [w228] mode=indexing
                    shift-right: [w226] -> _
                    shift-left: w224 -> [w227]
                    tunnel: [w225] -> w217 mode=indexing
                    n98 = call <vilib>:"DAQmx Start Task.vi"("task/channels in"=w228, "error in"=w227) -> ("task out"=w225:refnum<k21>, "error out"=w226:errorcluster)  [unwired: 12 in]
                  }
                }
              }
            }
          }
        }
        frame #5 {
          n99 = Absolute Value(x=w244) -> (abs(x)=w238:i32)
          n100 = Unbundle By Name(w230) -> ("Bulk Acq"=w229:bool)
          n101 = Unbundle By Name(w235) -> ("Xmit Ring"=w234:i32)
          n102 = Unbundle By Name(w230) -> ("Main Digitizer"=w233:T9, "Dig Config"=w232:T10)
          n103 = Not Equal To 0?(x=w234) -> (x != 0?=w239:bool)
          n104 = Not And(1:w239, 2:w229) -> (0:w240:bool)
          n105 = Select(t=w238, s=w243, f=w242) -> (s? t:f=w241:i32)
          n106 = case shown="True" w240 {
            tunnel: [_ w255] -> w245
            tunnel: w232 -> [_ w248]
            tunnel: w243 -> [_ w253]
            tunnel: w241 -> [_ w254]
            tunnel: w237 -> [_ w251]
            tunnel: [_ w250] -> w236
            tunnel: w230 -> [_ w249]
            tunnel: w233 -> [_ w247]
            tunnel: w231 -> [_ w246]
            frame False {
            }
            frame True {
              # "set up A/D card for sequence acquistion using parameters selected earlier"
              n107 = case shown="\"2 Chans w/ 2 Acqiris\", Default" w248 {
                tunnel: w254 -> [_ w427]
                tunnel: [_ w428] -> w252
                tunnel: w253 -> [_ w426]
                tunnel: w247 -> [_ w425]
                tunnel: w249 -> [_ w424]
                frame "Single channel", "2 Chans w/ 1 Acqiris" {
                }
                frame "2 Chans w/ 2 Acqiris", Default {
                  n108 = Unbundle By Name(w424) -> ("rf points per line"=w423:i32)
                  n109 = case shown="\"Acqiris Digitizer\", Default" w425 {
                    tunnel: [w433 w443 _] -> w428
                    tunnel: w423 -> [w432 w441 _]
                    tunnel: w427 -> [w431 w442 _]
                    tunnel: w426 -> [w430 w440 _]
                    tunnel: w424 -> [w429 w439 _]
                    frame "Acqiris Digitizer", Default {
                      n110 = disable-structure shown="Disabled" {
                        disable-tunnel: [w438 _] -> w433
                        disable-tunnel: w432 -> [w437 _]
                        disable-tunnel: w431 -> [w436 _]
                        disable-tunnel: w430 -> [w435 _]
                        disable-tunnel: w429 -> [w434 _]
                        frame Disabled {
                          n111 = call "ArmCratePrams.vi"("Arm trig Not?"=w435, "num lines"=w436, "rf pts"=w437, "Digitizer Settings"=w434) -> ("error out"=w438:errorcluster)  [unwired: 10 in, 1 out]
                        }
                        frame Enabled {
                        }
                      }
                    }
                    frame "NI Digitizer" {
                      n112 = call "NIArmCratePrams.vi"("Arm Trig Not?"=w440, "num lines"=w442, "rf pts"=w441, "Digitizer Settings"=w439) -> ("error out"=w443:errorcluster)  [unwired: 11 in]
                    }
                    frame "LeCroy", "AlazarTech" {
                    }
                  }
                }
              }
              n113 = case shown="\"Acqiris Digitizer\"" w247 {
                tunnel: [w261 w297 w314 _ _ _ _] -> w255
                tunnel: w252 -> [w260 w289 _ _ _ _ _]
                tunnel: w253 -> [w259 w301 w333 w360 w384 w401 _]
                tunnel: w254 -> [w258 w303 w330 w361 w381 w396 _]
                tunnel: w251 -> [_ _ w317 _ _ _ _]
                tunnel: [_ _ _ _ _ w397 _] -> w250
                tunnel: w248 -> [_ _ _ _ _ w402 _]
                tunnel: w249 -> [w256 w291 w312 w343 w370 w391 _]
                tunnel: w246 -> [_ _ w309 _ _ _ _]
                frame "Acqiris Digitizer" {
                  n114 = Unbundle By Name(w256) -> ("Digitizer ID Cluster.Acqiris/Alazar/SP ID"=w257:u32[])
                  n115 = disable-structure shown="Disabled" {
                    disable-tunnel: [w282 _] -> w261
                    disable-tunnel: w260 -> [w281 _]
                    disable-tunnel: w259 -> [w280 _]
                    disable-tunnel: w258 -> [w279 _]
                    disable-tunnel: w257 -> [w278 _]
                    disable-tunnel: w256 -> [w273 _]
                    frame Disabled {
                      # "arm trigger"
                      # "set up for sequence"
                      n116 = Unbundle By Name(w273) -> ("rf points per line"=w262:i32, "Voltage Scale"=w272:dbl)
                      n117 = Index Array(array=w278) -> (element=w270:u32)  [unwired: 1 in]
                      n118 = call <instrlib>:"Query Vertical Settings.vi"("Instrument ID"=w270, "Channel (1)"=1) -> ("dup Instrument ID"=w268:u32, "Coupling"=w266:T21, "error out"=w269:errorcluster, "Offset"=w271:dbl)  [unwired: 2 in, 2 out]
                      n119 = To Word Integer(number=w266) -> (16bit integer=w264:i16)
                      n120 = Decrement(x=w264) -> (x-1=w265:i16)
                      n121 = call <instrlib>:"Configure Memory Settings.vi"("error in (no error)"=w269, "Number of Samples (1000)"=w262, "Number of Segments (1)"=w279, "Instrument ID"=w268) -> ("error out"=w275:errorcluster, "dup Instrument ID"=w277:u32)  [unwired: 2 out]
                      n122 = Bundle("Voltage Scale"=w272, "Offset"=w271, w265) -> (w267:cluster{"Voltage Scale":dbl, "Offset":dbl, i16})  [unwired: 1 in]
                      n123 = call "conVert.vi"("InstrumentID"=w277, "V scale"=w267, "error in"=w275) -> ("Status"=w276:i32, "error out"=w274:errorcluster)  [unwired: 2 in, 1 out]
                      n124 = call "conSamp.vi"("error in"=w274, "Digitizer Settings"=w273, "InstrumentID"=w276) -> ("error out"=w283:errorcluster, "DUP ID"=w284:u32)  [unwired: 1 in]
                      n125 = case shown="False" w280 {
                        tunnel: w284 -> [w287 _]
                        tunnel: w283 -> [w286 w288]
                        tunnel: [w285 w288] -> w282
                        tunnel: w281 -> [_ _]
                        frame False {
                          n126 = call <instrlib>:"Start Acquisition.vi"("error in (no error)"=w286, "Instrument ID"=w287) -> ("error out"=w285:errorcluster)  [unwired: 2 in, 1 out]
                        }
                        frame True {
                        }
                      }
                    }
                    frame Enabled {
                    }
                  }
                }
                frame "NI Digitizer", Default {
                  n127 = Unbundle By Name(w291) -> ("Digitizer ID Cluster.NI Instr Handles"=w294:refnum<k15>[])
                  n128 = Unbundle By Name(w291) -> ("rf points per line"=w290:i32)
                  n129 = Unbundle By Name(w291) -> ("Voltage Scale"=w293:dbl)
                  n130 = Index Array(array=w294) -> (element=w295:refnum<k15>)  [unwired: 1 in]
                  n131 = property class="niScope"(reference=w295, "Reference Position"=0, "Min Number of Points"=w290, "Number of Records"=w303, "Enable Records > Memory"=TRUE, "Vertical Range"=w293) -> (reference out=w300:refnum<k15>, error out=w292:errorcluster)  [unwired: 1 in]
                  n132 = call "NI conSamp.vi"("error in"=w292, "Digitizer Settings"=w291, "InstrumentID"=w300) -> ("error out"=w298:errorcluster, "DUP ID"=w299:refnum<k15>)  [unwired: 1 in]
                  n133 = case shown="False" w301 {
                    tunnel: w299 -> [w306 _]
                    tunnel: w298 -> [w305 w307]
                    tunnel: [w304 w307] -> w297
                    tunnel: w289 -> [_ _]
                    frame False {
                      n134 = call <instrlib>:"niScope Initiate Acquisition.vi"("instrument handle"=w306, "error in"=w305) -> ("error out"=w304:errorcluster)  [unwired: 1 in, 12 out]
                    }
                    frame True {
                    }
                  }
                }
                frame "LeCroy" {
                  w320 = u16 0 items=["RealTime", "RIS", "Sequence", "Roll", "WaveStream"] ("Sample Mode (0: RealTime)")
                  w329 = FALSE ("Continuous Acquisition Mode (T: On)")
                  w319 = u16 2 items=["RealTime", "RIS", "Sequence", "Roll", "WaveStream"] ("Sample Mode (0: RealTime)")
                  # "Need delay first time due to lag in LeCroy"
                  n135 = Unbundle By Name(w312) -> ("Digitizer delay (us)"=w313:dbl)
                  n136 = Unbundle By Name(w312) -> ("Digitizer ID Cluster.LeCroy VISA"=w311:refnum<visa-resource-name>)
                  n137 = call <instrlib>:"Configure Continuous Acquisition.vi"("Auto Trigger Enabled (T: Normal)"=w329, "Continuous Acquisition Mode (T: On)"=w329, "VISA resource name"=w311) -> ("error out"=w331:errorcluster, "VISA resource name out"=w332:refnum<visa-resource-name>)  [unwired: 7 in]
                  n138 = Equal?(x=-1 ("y"), y=w317) -> (x = y?=w310:bool)
                  n139 = expression code="-1E-6*x"(w313) -> (w327:dbl)
                  n140 = Select(t=w320, s=w310, f=w319) -> (s? t:f=w318:u16)
                  n141 = Number To Exponential String(number=w327) -> (E-format string=w328:string)  [unwired: 3 in]
                  n142 = call <instrlib>:"Configure Sample Mode.vi"("error in (no error)"=w331, "Number of Segments (2)"=w330, "Sample Mode (0: RealTime)"=w318, "VISA resource name"=w332) -> ("error out"=w325:errorcluster, "VISA resource name out"=w326:refnum<visa-resource-name>)  [unwired: 6 in]
                  n143 = Concatenate Strings("TRDL " ("Write Buffer"), w328) -> (w324:string)
                  n144 = call <instrlib>:"Write.vi"("error in (no error)"=w325, "Write Buffer"=w324, "VISA resource name"=w326) -> ("error out"=w322:errorcluster, "VISA resource name out"=w321:refnum<visa-resource-name>)  [unwired: 6 in, 1 out]
                  n145 = case shown="False" w333 {
                    tunnel: w321 -> [w339 _]
                    tunnel: w322 -> [w338 w340]
                    tunnel: [w337 w340] -> w315
                    frame False {
                      n146 = call <instrlib>:"Initiate.vi"("error in (no error)"=w338, "VISA resource name"=w339) -> ("error out"=w337:errorcluster)  [unwired: 8 in, 1 out]
                    }
                    frame True {
                    }
                  }
                  n147 = Unbundle By Name(w309) -> ("Plane"=w308:i32)
                  n148 = case shown="0" w308 {
                    tunnel: w315 -> [w334 w336]
                    tunnel: [w334 w336] -> w314
                    frame 0 {
                      n149 = Wait (ms)(milliseconds to wait=500) -> ()  [unwired: 1 out]
                    }
                    frame 1, Default {
                    }
                  }
                }
                frame "GaGe" {
                  w356 = 128
                  # "might need to update samp rate in but should occur only if predefined samp freqs are wrong"
                  # "USB version with no delay support. Must take too many pts"
                  n150 = Unbundle By Name(w343) -> ("rf points per line"=w341:i32, "Samp Rate (Hz)"=w345:dbl, "Digitizer delay (us)"=w346:dbl, "Additional dig delay (us)"=w347:dbl, "Offset delay (us)"=w348:dbl)
                  n151 = Unbundle By Name(w343) -> ("Digitizer ID Cluster.GaGe Handle"=w342:T22)
                  n152 = Compound Arithmetic op=ADD(w346, w347, w348) -> (w344:dbl)
                  n153 = Multiply(x=w345, y=w344) -> (x*y=w352:dbl)
                  n154 = expression code="x*1E-6"(w352) -> (w351:dbl)
                  n155 = Add(x=w341, y=w351) -> (x+y=w354:dbl)
                  n156 = Quotient & Remainder(x=w354, y=w356) -> (floor(x/y)=w355:dbl)  [unwired: 1 out]
                  n157 = Increment(x=w355) -> (x+1=w357:dbl)
                  n158 = Multiply(x=w357, y=w356) -> (x*y=w353:dbl)
                  n159 = Bundle(cluster=T17 {0.0, "Clock mode"=enum."Internal", "RingText.Text"="Single", 0, 0, "time out (ms)"=0.0, 0.0, 0.0} ("output cluster"), w345, w353, w353) -> (w362:T17)  [unwired: 5 in]
                  n160 = call "CsTool-ConfigureAcquisitionAll.vi"("Handle Cluster"=w342, "Segment Count (1)"=w361, "Acquisition"=w362) -> ("Error Code"=w358:i32)  [unwired: 2 in]
                  n161 = flat-sequence {
                    tunnel: [w365] -> w359
                    tunnel: w342 -> [w365]
                    tunnel: [w366] -> _
                    tunnel: w358 -> [_]
                    tunnel: [w365] -> w350
                    frame #0 {
                      w367 = TRUE
                      n162 = call "CsTool-CommitAll.vi"("OnlyOnChange (t)"=w367, "Coerce Flag (f)"=w367, "Handle Cluster"=w365) -> ("Error Code"=w366:i32)  [unwired: 1 out]
                    }
                  }
                  n163 = call "CsTool-QueryAcquisitionParametersFill.vi"("Handle Cluster"=w350) -> ("Sample Rate"=w349:dbl)  [unwired: 10 out]
                  n164 = case shown="False" w360 {
                    tunnel: w359 -> [w364 _]
                    frame False {
                      n165 = call "CsTool-CaptureFill.vi"("Handle Cluster"=w364) -> ()  [unwired: 1 out]
                    }
                    frame True {
                    }
                  }
                  n166 = Bundle By Name(cluster=w343, "Samp Rate (Hz)"=w349) -> ()  [unwired: 1 out]
                }
                frame "Teledyne" {
                  # "extra shift needed to hit delay"
                  # "might need to update samp rate in but should occur only if predefined samp freqs are wrong"
                  n167 = Unbundle By Name(w370) -> ("Digitizer ID Cluster.ADQRef"=w375:refnum<k24>, "Digitizer ID Cluster.adq_cu_ptr"=w373:refnum<k24>, "Digitizer ID Cluster.GaGe Handle.Boards"=w372:u32)
                  n168 = Unbundle By Name(w370) -> ("rf points per line"=w369:i32)
                  n169 = call "DelayPtsAdjust.vi"("CalcPt?"=TRUE, "Digitizer Settings"=w370) -> ("Actual Delay pts"=w376:u32, "PostDelayCorrection"=w377:u32)  [unwired: 8 in]
                  n170 = call "SPADQ_DisarmArmTrigger.vi"("adq_num"=w372, "adq_cu_ptr in"=w373, "ADQAPI Ref"=w375) -> ("error out"=w368:errorcluster, "ADQAPI Ref (out)"=w374:refnum<k24>)  [unwired: 7 in]
                  n171 = call "SPADQ_TrigDelay.vi"("Delay in Pts"=w376, "error in (no error)"=w368, "adq_num"=w372, "adq_cu_ptr in"=w373, "ADQAPI Ref"=w374) -> ("error out"=w382:errorcluster, "ADQAPI Ref (out)"=w383:refnum<k24>)  [unwired: 4 in, 1 out]
                  n172 = Add(x=w377, y=w369) -> (x+y=w380:u32)
                  n173 = call "SPADQ_MultiRecord.vi"("Records"=w381, "Pts to Acquire"=w380, "error in (no error)"=w382, "adq_num"=w372, "adq_cu_ptr in"=w373, "ADQAPI Ref"=w383) -> ("error out"=w378:errorcluster, "ADQAPI Ref (out)"=w379:refnum<k24>)  [unwired: 3 in, 1 out]
                  n174 = case shown="False" w384 {
                    tunnel: w379 -> [w386 _]
                    tunnel: w378 -> [w385 _]
                    tunnel: w373 -> [w387 _]
                    tunnel: w372 -> [w388 _]
                    frame False {
                      n175 = call "SPADQ_ArmTrigger.vi"("error in (no error)"=w385, "adq_num"=w388, "adq_cu_ptr in"=w387, "ADQAPI Ref"=w386) -> ()  [unwired: 6 in, 2 out]
                    }
                    frame True {
                    }
                  }
                }
                frame "AlazarTech" {
                  w398 = u16 2 items=["DC 1 MOhm", "AC 1 MOhm", "DC 50 Ohm", "AC 50 OHM"] ("Crate Coupling")
                  # "Delay in pts"
                  n176 = Unbundle By Name(w391) -> ("Digitizer ID Cluster.Acqiris/Alazar/SP ID"=w392:u32[], "Voltage Scale"=w400:dbl)
                  n177 = Unbundle By Name(w391) -> ("Digitizer ID Cluster.GaGe Handle.Boards"=w389:u32, "rf points per line"=w390:i32)
                  n178 = case shown="\"2 Chans w/ 2 Acqiris\", Default" w402 {
                    tunnel: [w415 w417] -> w394
                    tunnel: w389 -> [_ w416]
                    frame "Single channel" {
                      w415 = u32 1 items=["A"=1, "B"=2, "A + B"=3, "C"=4, "A + C"=5, "A + B"=6, "D"=8, "A + D"=9, "B + D"=10, "C + D"=12, "A + B + C + D"=15] ("Channel")
                    }
                    frame "2 Chans w/ 2 Acqiris", Default {
                      n179 = case shown="16" w416 {
                        tunnel: [w418 w419] -> w417
                        frame 2, Default {
                          w418 = u32 3 items=["A"=1, "B"=2, "A + B"=3, "C"=4, "A + C"=5, "A + B"=6, "D"=8, "A + D"=9, "B + D"=10, "C + D"=12, "A + B + C + D"=15] ("Channel")
                        }
                        frame 16 {
                          w419 = u32 15 items=["A"=1, "B"=2, "A + B"=3, "C"=4, "A + C"=5, "A + B"=6, "D"=8, "A + D"=9, "B + D"=10, "C + D"=12, "A + B + C + D"=15] ("Channel")
                        }
                      }
                    }
                  }
                  n180 = Bundle("Voltage Scale"=w400, "Voltage Scale"=0.0, "Crate Coupling"=w398) -> (w395:T23)  [unwired: 1 out]
                  n181 = for {
                    tunnel: [w414] -> w397
                    tunnel: w391 -> [w413]
                    tunnel: w396 -> [w411]
                    tunnel: w390 -> [w409]
                    tunnel: w395 -> [w406]
                    tunnel: w392 -> [w405] mode=indexing
                    tunnel: w394 -> [w403]
                    tunnel: [w404] -> w393
                    n182 = call "Alazar_ChannelConfig - ATS-SDK.vi"("V scale"=w406, "Channel"=w403, "Handle in"=w405) -> ("error out"=w407:errorcluster, "Handle_Out"=w408:u32)  [unwired: 2 in, 1 out]
                    n183 = call "AlazarAcqPrep - ATS-SDK.vi"("Handle"=w408, "Digitizer Settings"=w413, "Enable Trigger Enable"=FALSE, "Channel"=w403, "BuffCount"=2, "rf points per line"=w409, "error in (no error)"=w407, "rf lines per buffer"=w411) -> ("AlazarCluster"=w414:T24, "error out"=w404:errorcluster)  [unwired: 4 in, 2 out]
                  }
                  n184 = case shown="False" w401 {
                    tunnel: w393 -> [w422 _]
                    tunnel: w392 -> [w421 _]
                    frame False {
                      n185 = Index Array(array=w421) -> (element=w420:u32)  [unwired: 1 in]
                      n186 = call "AlazarStartCapture.vi"("Handle"=w420, "error in (no error)"=w422) -> ()  [unwired: 3 out]
                    }
                    frame True {
                    }
                  }
                }
                frame "No Digitizer" {
                }
              }
            }
          }
        }
        frame #6 {
          # "start counters, scope will start taking data unless motor needs\nto move. Acquistion start when prf counter start or when motor starts to move"
          n187 = Not(x=w450) -> (.not. x?=w449:bool)
          n188 = And(x=w449, y=w451) -> (x .and. y?=w446:bool)
          n189 = case shown="\"Therapy With Scan\", Default" w447 {
            tunnel: [_ TRUE] -> w445
            frame "Therapy With Scan", Default {
            }
            frame "1-D B-Scan PRF", "2-D B-Scan PRF" {
            }
          }
          n190 = Compound Arithmetic op=OR(w454, w453, w446, w445) -> (w452:bool)
          n191 = case shown="True" w452 {
            tunnel: w455 -> [_ w460]
            tunnel: w444 -> [_ w459]
            frame False {
            }
            frame True {
              n192 = case shown="\"SERI GP\"" w459 {
                tunnel: w460 -> [w461 _]
                frame "WCM Main", Default {
                  n193 = call <vilib>:"DAQmx Start Task.vi"("task/channels in"=w461) -> ()  [unwired: 1 in, 14 out]
                }
                frame "SERI GP" {
                }
              }
            }
          }
          n194 = case shown="True" w448 {
            frame False {
            }
            frame True {
              w458 = refnum<k21> "Dev2 Gate"  # DAQmx Task Name
              n195 = call-poly <vilib>:"DAQmx Write.vi"("task/channels in"=w458, "data"=TRUE) -> ()  [unwired: 11 in, 3 out]
            }
          }
        }
        frame #7 {
          # "Turn on PRF source"
          # "move motor if needed or move on"
          n196 = case shown="False" w477 {
            tunnel: w476 -> [_ w518]
            tunnel: w474 -> [_ w517]
            tunnel: w475 -> [_ w516]
            tunnel: w473 -> [_ w515]
            tunnel: w472 -> [_ w514]
            tunnel: w471 -> [w480 _]
            tunnel: w469 -> [_ w513]
            tunnel: w470 -> [_ w512]
            tunnel: w468 -> [_ w511]
            tunnel: w467 -> [_ w509]
            tunnel: w466 -> [_ w508]
            tunnel: w465 -> [w479 _]
            tunnel: w464 -> [_ w507]
            tunnel: w463 -> [_ w506]
            tunnel: w462 -> [w478 w505]
            frame False {
              n197 = case shown="\"WCM Main\", Default" w480 {
                tunnel: w479 -> [w484 _ _ _]
                tunnel: w478 -> [w482 w488 _ w498]
                frame "WCM Main", Default {
                  # "use function generator pr or internal ctr prf"
                  n198 = case shown="False" w484 {
                    tunnel: [w485 w486] -> w483
                    frame False {
                      w485 = u16 0 items=["Function Gen Input", "Motion Trig", "Internal RT Motion Trig", "Internal CTR 1 Output"] ("Trig Source")
                    }
                    frame True {
                      w486 = u16 3 items=["Function Gen Input", "Motion Trig", "Internal RT Motion Trig", "Internal CTR 1 Output"] ("Trig Source")
                    }
                  }
                  n199 = Unbundle By Name(w482) -> ("GL Ref Out"=w481:refnum<k7>)
                  n200 = call "RouteTrigSource.vi"("Galil.IGalil"=w481, "Trig Source"=w483) -> ()  [unwired: 9 in, 1 out]
                }
                frame "Hawaii", "SERI GP" {
                  # "Use BreakPt PRF"
                  n201 = Unbundle By Name(w488) -> ("Motion System"=w487:T5)
                  n202 = case shown="\"Galil\"" w487 {
                    tunnel: w488 -> [_ w489 w496]
                    frame "MM3000", Default {
                    }
                    frame "NI 735x" {
                      n203 = disable-structure shown="Disabled" {
                        disable-tunnel: w489 -> [w491 _]
                        frame Disabled {
                          n204 = Unbundle By Name(w491) -> ("Motion Bd ID"=w490:u8)
                          n205 = call <vilib>:"Run Program.flx"("Program (1)"=3, "Board ID"=w490) -> ()  [unwired: 1 in, 6 out]
                        }
                        frame Enabled {
                        }
                      }
                    }
                    frame "Galil" {
                      n206 = Unbundle By Name(w496) -> ("GL Ref Out"=w495:refnum<k7>)
                      n207 = call "GL Command Set.vi"("Command"=Command_Menu."Execute", "Text Input"="#PRF", "Galil.IGalil"=w495) -> ()  [unwired: 4 in, 5 out]
                    }
                  }
                }
                frame "Columbia MM3000" {
                  (unwired) "SB3"
                  # "Old send command mm2k"
                }
                frame "UHI Allen" {
                  n208 = Unbundle By Name(w498) -> ("ESP VISA"=w497:refnum<visa-resource-name>)
                  n209 = call <instrlib>:"Get DIO Port AB Bit Status.vi"("VISA resource name"=w497) -> ("error out"=w500:errorcluster, "DIO Port A status"=w503:T25, "VISA resource name out"=w499:refnum<visa-resource-name>)  [unwired: 4 in]
                  n210 = Bundle By Name(cluster=w503, "Port A bit-1 at logic level"=FALSE) -> (w501:T25)
                  n211 = call <instrlib>:"Set DIO Port AB Bit Status.vi"("error in (no error)"=w500, "DIO Port status"=w501, "VISA resource name"=w499) -> ()  [unwired: 3 in, 2 out]
                }
              }
            }
            frame True {
              n212 = Unbundle By Name(w505) -> ("Motion System"=w504:T5)
              n213 = case shown="\"NI 735x\", Default" w504 {
                tunnel: w518 -> [_ w531 w556 _]
                tunnel: w517 -> [_ w530 w555 _]
                tunnel: w516 -> [_ w529 w554 _]
                tunnel: w515 -> [_ w528 w549 _]
                tunnel: "start value" -> [_ w527 w553 _]
                tunnel: w514 -> [_ w526 w552 _]
                tunnel: w513 -> [_ w525 w551 _]
                tunnel: w512 -> [_ w524 _ _]
                tunnel: w511 -> [_ w523 w550 _]
                tunnel: w509 -> [_ w522 _ _]
                tunnel: w508 -> [_ _ _ w558]
                tunnel: w507 -> [_ w521 _ _]
                tunnel: w506 -> [_ w520 w548 _]
                tunnel: w505 -> [_ w519 w547 _]
                frame "MM3000" {
                }
                frame "NI 735x", Default {
                  n214 = case shown="0" w524 {
                    tunnel: w531 -> [w542 _ _]
                    tunnel: w530 -> [w541 _ _]
                    tunnel: w529 -> [w540 _ _]
                    tunnel: w528 -> [w539 _ _]
                    tunnel: w527 -> [w538 _ _]
                    tunnel: w526 -> [w537 _ _]
                    tunnel: w525 -> [w536 _ _]
                    tunnel: w523 -> [w535 _ _]
                    tunnel: w522 -> [_ w543 w545]
                    tunnel: [_ w544 _] -> _
                    tunnel: w521 -> [w534 _ _]
                    tunnel: w520 -> [w533 _ _]
                    tunnel: w519 -> [w532 _ _]
                    frame 0 {
                      # "move motor down axis"
                      n215 = call "PerformScan.vi"("Avg Num Mod"=w539, "Therapy/AVG ?"=w541, "AlazarCluster"=w534, "Line Axis"=w540, "Type of scan"=w537, "lines per scan plane mod"=w536, "Reverse ?"=w542, "Digitizer Settings"=w533, "Motion Settings In"=w532, "File Names"=w535, "Offset"=w538) -> ()  [unwired: 5 in]
                    }
                    frame 1, Default {
                      # "External EKG signal."
                      n216 = call <vilib>:"DAQmx Start Task.vi"("task/channels in"=w543) -> ("error out"=w544:errorcluster)  [unwired: 13 in, 1 out]
                    }
                    frame 2 {
                      # "Orlando drops IQ vi here which starts CTR1"
                      n217 = call <vilib>:"DAQmx Start Task.vi"("task/channels in"=w545) -> ()  [unwired: 1 in, 14 out]
                    }
                  }
                }
                frame "Newport ESP" {
                  n218 = Unbundle By Name(w547) -> ("ESP VISA"=w546:refnum<visa-resource-name>)
                  n219 = call "PerformScan_ESP.vi"("ESP VISA"=w546, "Therapy/AVG ?"=w555, "Motion Settings"=w547, "Line Axis"=w554, "Type of scan"=w552, "lines per scan plane"=w551, "Reverse ?"=w556, "Avg Num"=w549, "Digitizer Settings"=w548, "File Names"=w550, "Offset"=w553) -> ()  [unwired: 4 in, 1 out]
                }
                frame "No Motion Card" {
                  (unwired) FALSE
                  n220 = call-poly <vilib>:"DAQmx Write.vi"("task/channels in"=w558, "data"=TRUE ("stop (T)")) -> ()  [unwired: 11 in, 3 out]
                }
              }
            }
          }
        }
        frame #8 {
          n221 = case shown="1" w564 {
            tunnel: w566 -> [w570 w581]
            tunnel: [FALSE w579] -> w565
            tunnel: [w570 w576] -> w559
            tunnel: w563 -> [_ w578]
            tunnel: w561 -> [_ w572]
            tunnel: w562 -> [_ w574]
            frame 0, Default {
            }
            frame 1 {
              # "Check to see if data acquistion is finished. WaitTWO seconds more and then force extra trigs if needed. Data should all be taken be the time this frame is reached. May need more sophisticated error checking"
              n222 = Unbundle By Name(w572) -> ("Main Digitizer"=w571:T9, "DigTimeOut"=w573:sgl)
              n223 = expression code="x*1000"(w573) -> (w575:sgl)
              n224 = case shown="\"Acqiris Digitizer\"" w571 {
                tunnel: w581 -> [w588 w608 w614 w620 _ _]
                tunnel: w578 -> [w584 _ _ _ _ _]
                tunnel: [w585 w608 w614 w619 _ _] -> w576
                tunnel: [w587 _ _ _ _ _] -> w580
                tunnel: [w586 _ _ _ _ _] -> w577
                tunnel: w575 -> [w583 _ w609 w618 w624 _]
                tunnel: w574 -> [_ _ _ w617 _ _]
                tunnel: w572 -> [w582 _ w613 w616 w621 _]
                frame "Acqiris Digitizer" {
                  n225 = disable-structure shown="Disabled" {
                    disable-tunnel: w588 -> [w599 _]
                    disable-tunnel: [w598 _] -> w587
                    disable-tunnel: [w596 _] -> w586
                    disable-tunnel: [w595 _] -> w585
                    disable-tunnel: w584 -> [w594 _]
                    disable-tunnel: w583 -> [w593 _]
                    disable-tunnel: w582 -> [w590 _]
                    frame Disabled {
                      n226 = Unbundle By Name(w590) -> ("Digitizer ID Cluster.Acqiris/Alazar/SP ID"=w591:u32[])
                      n227 = Index Array(array=w591) -> (element=w592:u32)  [unwired: 1 in]
                      n228 = call "WaitForSegs.vi"("Acqiris ID"=w592, "lines per plane"=w594, "error in"=w599, "Timeout"=w593) -> ("status"=w598:bool, "error out"=w597:errorcluster)  [unwired: 2 out]
                      n229 = Unbundle By Name(w590) -> ("Dig Config"=w589:T10)
                      n230 = case shown="\"2 Chans w/ 2 Acqiris\"" w589 {
                        tunnel: w594 -> [_ w607]
                        tunnel: w597 -> [w600 w606]
                        tunnel: [w600 w605] -> w595
                        tunnel: [_ w604] -> w596
                        tunnel: w591 -> [_ w603]
                        frame "Single channel", Default {
                        }
                        frame "2 Chans w/ 2 Acqiris" {
                          n231 = Index Array(array=w603, index=1) -> (element=w602:u32)
                          n232 = call "WaitForSegs.vi"("Acqiris ID"=w602, "lines per plane"=w607, "error in"=w606) -> ("status"=w604:bool, "error out"=w605:errorcluster)  [unwired: 1 in, 2 out]
                        }
                      }
                    }
                    frame Enabled {
                    }
                  }
                }
                frame "NI Digitizer", Default {
                }
                frame "Teledyne" {
                  n233 = Unbundle By Name(w613) -> ("Digitizer ID Cluster.ADQRef"=w612:refnum<k24>, "Digitizer ID Cluster.adq_cu_ptr"=w611:refnum<k24>, "Digitizer ID Cluster.GaGe Handle.Boards"=w610:u32)
                  n234 = call "SPADQ_AcquisitionStatus.vi"("WaitTime (ms)"=w609, "adq_num"=w610, "adq_cu_ptr in"=w611, "ADQAPI Ref"=w612) -> ()  [unwired: 4 in, 4 out]
                }
                frame "LeCroy" {
                  n235 = Unbundle By Name(w616) -> ("Digitizer ID Cluster.LeCroy VISA"=w615:refnum<visa-resource-name>)
                  n236 = call "TimeOut+ForceTrigger.vi"("error in (no error)"=w620, "lines per plane mod"=w617, "Timeout (10000 ms)"=w618, "VISA resource name"=w615) -> ("error out"=w619:errorcluster)  [unwired: 4 in, 3 out]
                }
                frame "GaGe" {
                  n237 = Unbundle By Name(w621) -> ("Digitizer ID Cluster.GaGe Handle"=w622:T22)
                  n238 = expression code="x/1000"(w624) -> (w623:sgl)
                  n239 = call "GaGe_TimeoutFill.vi"("TimeOut (s)"=w623, "GaGe Handle"=w622) -> ()  [unwired: 8 in, 2 out]
                }
                frame "AlazarTech" {
                }
              }
              n240 = Or(x=w577, y=w580) -> (x .or. y?=w579:bool)
            }
          }
          n241 = case shown="True" w560 {
            frame False {
            }
            frame True {
              w568 = refnum<k21> "Dev2 Gate"  # DAQmx Task Name
              n242 = call-poly <vilib>:"DAQmx Write.vi"("task/channels in"=w568, "data"=FALSE) -> ()  [unwired: 11 in, 3 out]
            }
          }
        }
        frame #9 {
          # "get data from scope, as 8 bit integers."
          n243 = case shown="True" w631 {
            tunnel: w635 -> [_ w650]
            tunnel: w634 -> [_ w647]
            tunnel: w633 -> [_ w649]
            tunnel: w632 -> [_ w645]
            tunnel: w630 -> [_ w643]
            tunnel: w629 -> [_ w642]
            tunnel: w628 -> [_ w638]
            tunnel: w627 -> [_ w636]
            tunnel: w626 -> [_ w641]
            tunnel: w625 -> [_ w639]
            frame False {
            }
            frame True {
              # "Read data for array during next pass. Need to reduce index by one and not the reverse value. Test case for bulk acq mode"
              # "Don't reverse data if EKG Trig"
              n244 = Unbundle By Name(w641) -> ("Xmit Ring"=w640:i32)
              n245 = Unbundle By Name(w638) -> ("Dig Config"=w637:T10)
              n246 = Not Equal To 0?(x=w645) -> (x != 0?=w644:bool)
              n247 = Select(t=FALSE, s=w644, f=w647) -> (s? t:f=w646:bool)
              n248 = case shown="1, Default" w640 {
                selector: w640 -> [_ w667]
                tunnel: w650 -> [_ w669]
                tunnel: w649 -> [_ w668]
                tunnel: w646 -> [_ w665]
                tunnel: w643 -> [_ w661]
                tunnel: w642 -> [_ w660]
                tunnel: w638 -> [_ w659]
                tunnel: w638 -> [_ w658]
                tunnel: w641 -> [_ w655]
                tunnel: w639 -> [_ w654]
                tunnel: w637 -> [_ w653]
                tunnel: w636 -> [_ w651]
                frame 0 {
                }
                frame 1, Default {
                  n249 = Unbundle By Name(w658) -> ("Bulk Start Indexes"=w657:i32[], "Total Dig CH"=w656:i32)
                  n250 = Decrement(x=w667) -> (x-1=w662:i32)
                  n251 = Unbundle By Name(w651) -> ("Plane"=w652:i32)
                  n252 = call "FileNames.vi"("# Elements"=w656, "Plane"=w652, "Dig Config"=w653, "Xmit Ring"=w662, "Scan Name"=w660, "2-D motor"=w661) -> ("All files"=w663:string[])  [unwired: 1 in, 4 out]
                  n253 = Not(x=w665) -> (.not. x?=w664:bool)
                  n254 = Index Array(array=w657, index=w662) -> (element=w666:i32)
                  n255 = call "GetData.vi"("Digitizer Settings"=w659, "Ann Array Params"=w655, "Motion Settings"=w651, "All files"=w663, "error in"=w669, "lines per plane mod"=w668, "Type of scan"=w654, "Start Record"=w666, "Reverse ?"=w664) -> ()  [unwired: 8 in, 3 out]
                }
              }
            }
          }
        }
        frame #10 {
          # "get data from scope, as 8 bit integers."
          n256 = case shown="1" w675 {
            tunnel: w682 -> [_ w703]
            tunnel: w681 -> [_ w700]
            tunnel: w680 -> [_ w702]
            tunnel: w679 -> [_ w696]
            tunnel: w678 -> [_ w699]
            tunnel: w677 -> [_ w697]
            tunnel: w676 -> [_ w692]
            tunnel: w674 -> [_ w691]
            tunnel: w673 -> [_ w689]
            tunnel: w672 -> [_ w690]
            tunnel: w671 -> [_ w685]
            tunnel: w670 -> [_ w684]
            frame 0, Default {
            }
            frame 1 {
              # "Don't reverse data if EKG Trig"
              n257 = Unbundle By Name(w685) -> ("Xmit Ring"=w686:i32)
              n258 = Unbundle By Name(w689) -> ("Total Dig CH"=w688:i32, "Bulk Acq"=w683:bool)
              n259 = Decrement(x=w688) -> (x-1=w687:i32)
              n260 = Not Equal To 0?(x=w696) -> (x != 0?=w695:bool)
              n261 = Not Equal?(x=w686, y=w687) -> (x != y?=w693:bool)
              n262 = Select(t=FALSE, s=w695, f=w700) -> (s? t:f=w698:bool)
              n263 = Not And(1:w693, 2:w683) -> (0:w694:bool)
              n264 = case shown="True" w694 {
                tunnel: w703 -> [_ w745]
                tunnel: w702 -> [_ w744]
                tunnel: w699 -> [_ w743]
                tunnel: w698 -> [_ w741]
                tunnel: w697 -> [w708 _]
                tunnel: w692 -> [_ w739]
                tunnel: w691 -> [_ w737]
                tunnel: w689 -> [_ w735]
                tunnel: w690 -> [w705 w736]
                tunnel: w685 -> [_ w732]
                tunnel: w687 -> [_ w733]
                tunnel: w684 -> [_ w730]
                frame False {
                  n265 = flat-sequence {
                    tunnel: w708 -> [w712]
                    tunnel: [w712] -> w707
                    tunnel: [w710] -> w706
                    tunnel: w705 -> [w710]
                    tunnel: [w709] -> w704
                    tunnel: w707 -> [w716]
                    tunnel: [w715] -> _
                    tunnel: w706 -> [w714]
                    tunnel: w704 -> [w713]
                    frame #0 {
                      n266 = Unbundle By Name(w710) -> ("Motion System"=w709:T5)
                      n267 = Wait (ms)(milliseconds to wait=35) -> ()  [unwired: 1 out]
                    }
                    frame #1 {
                      n268 = case shown="\"NI 735x\"" w713 {
                        tunnel: w716 -> [_ w719 w724]
                        tunnel: [_ w717 w723] -> w715
                        tunnel: w714 -> [_ w721 w722]
                        frame "MM3000", Default {
                        }
                        frame "Galil" {
                          n269 = Unbundle By Name(w721) -> ("GL Ref Out"=w720:refnum<k7>)
                          n270 = Decrement(x=w719) -> (x-1=w718:i32)
                          n271 = call "GL CheckForMotion.vi"("Axis"=w718, "Refnum in"=w720) -> ("error out"=w717:errorcluster)  [unwired: 7 in, 2 out]
                        }
                        frame "NI 735x" {
                          n272 = disable-structure shown="Disabled" {
                            disable-tunnel: w724 -> [w729 _]
                            disable-tunnel: [w727 _] -> w723
                            disable-tunnel: w722 -> [w726 _]
                            frame Disabled {
                              n273 = Unbundle By Name(w726) -> ("Motion Bd ID"=w725:u8)
                              n274 = call-poly <vilib>:"Wait for Move Complete.flx"("Poll Interval (20 ms)"=3, "Axis or Vector Space"=w729, "Board ID"=w725) -> ("error out"=w727:errorcluster)  [unwired: 3 in, 5 out]
                            }
                            frame Enabled {
                            }
                          }
                        }
                      }
                    }
                  }
                }
                frame True {
                  n275 = Unbundle By Name(w735) -> ("Bulk Start Indexes"=w734:i32[])
                  n276 = case shown="True" w739 {
                    tunnel: w734 -> [_ w749]
                    tunnel: [0 w748] -> w738
                    tunnel: w733 -> [_ w747]
                    frame False {
                    }
                    frame True {
                      n277 = Index Array(array=w749, index=w747) -> (element=w748:i32)
                    }
                  }
                  n278 = Unbundle By Name(w732) -> ("Synth Foc?"=w731:bool)
                  n279 = Not(x=w731) -> (.not. x?=w740:bool)
                  n280 = call "GetData.vi"("AlazarCluster"=w737, "Digitizer Settings"=w735, "Ann Array Params"=w732, "Motion Settings"=w736, "All files"=w743, "error in"=w745, "lines per plane mod"=w744, "Type of scan"=w730, "save?"=w740, "Start Record"=w738, "Reverse ?"=w741) -> ("error out"=→"error out":errorcluster)  [unwired: 6 in, 2 out]
                }
              }
            }
          }
        }
        frame #11 {
          # "Shift to new pulse channel after scan and before data transfer."
          n281 = Unbundle By Name(w752) -> ("Xmit Ring"=w751:i32)
          n282 = global read "SwitchGlobals.vi" "Switch Unit"() -> (w753:T26)
          n283 = case shown="True" w754 {
            tunnel: w751 -> [_ w758]
            tunnel: w753 -> [_ w757]
            tunnel: w750 -> [_ w756]
            frame False {
            }
            frame True {
              n284 = Unbundle By Name(w756) -> ("Dig Config"=w755:T10)
              n285 = case shown="\"Single channel\"" w755 {
                tunnel: w758 -> [_ w760]
                tunnel: w757 -> [_ w761]
                frame "Single channel" {
                }
                frame "2 Chans w/ 2 Acqiris", Default {
                  n286 = Increment(x=w760) -> (x+1=w759:i32)
                  n287 = Increment(x=w759) -> (x+1=w762:i32)
                  n288 = case shown="\"Pickering\"" w761 {
                    tunnel: w762 -> [w763 w766 _]
                    frame "Cytex", Default {
                      n289 = case shown="0, Default" w763 {
                        selector: w763 -> [w764 _]
                        frame 0, Default {
                          n290 = call "Cytex.vi"("Xmit Ring"=w764) -> ()  [unwired: 2 in, 3 out]
                        }
                        frame 6 {
                          n291 = call "Cytex.vi"("Xmit Ring"=1) -> ()  [unwired: 2 in, 3 out]
                        }
                      }
                    }
                    frame "Pickering" {
                      n292 = disable-structure shown="Disabled" {
                        disable-tunnel: w766 -> [w767 _]
                        frame Disabled {
                          n293 = case shown="6" w767 {
                            selector: w767 -> [w768 _]
                            frame 0, Default {
                              n294 = call "PickeringBlank.vi"("Xmit Ring"=w768) -> ()  [unwired: 5 out]
                            }
                            frame 6 {
                              n295 = call "PickeringBlank.vi"("Xmit Ring"=1) -> ()  [unwired: 5 out]
                            }
                          }
                        }
                        frame Enabled {
                        }
                      }
                    }
                    frame "No Switch" {
                    }
                  }
                }
              }
            }
          }
        }
        frame #12 {
          n296 = case shown="\"1-D B-Scan PRF\", \"2-D B-Scan PRF\"" w774 {
            tunnel: [_ TRUE] -> w773
            frame "Therapy With Scan", Default {
            }
            frame "1-D B-Scan PRF", "2-D B-Scan PRF" {
            }
          }
          n297 = Not(x=w776) -> (.not. x?=w775:bool)
          n298 = And(x=w775, y=w778) -> (x .and. y?=w777:bool)
          n299 = Not Equal To 0?(x=w782) -> (x != 0?=w781:bool)
          n300 = Compound Arithmetic op=OR(w771, w779, w781, w777, w773) -> (w780:bool)
          n301 = case shown="True" w780 {
            tunnel: w783 -> [_ w791]
            tunnel: [_ w790] -> _
            tunnel: w772 -> [_ w788]
            tunnel: w770 -> [_ w787]
            frame False {
            }
            frame True {
              w789 = u16 1 items=["Function Gen Input", "Motion Trig", "Internal RT Motion Trig", "Internal CTR 1 Output"] ("Trig Source")
              # "stop counters again"
              n302 = Unbundle By Name(w788) -> ("GL Ref Out"=w786:refnum<k7>)
              n303 = call "RouteTrigSource.vi"("Galil.IGalil"=w786, "Trig Source"=w789) -> ("error out"=w785:errorcluster)  [unwired: 9 in]
              n304 = case shown="\"SERI GP\"" w787 {
                tunnel: w791 -> [_ w799]
                tunnel: [w792 w798] -> w790
                tunnel: w786 -> [w794 _]
                tunnel: w785 -> [w793 w797]
                frame "SERI GP" {
                  n305 = call "GL Command Set.vi"("Command"=Command_Menu."Halt Execute", "error in (no error)"=w793, "Value"=-1, "Galil.IGalil"=w794) -> ("error out"=w792:errorcluster)  [unwired: 3 in, 4 out]
                }
                frame "WCM Main", Default {
                  n306 = call <vilib>:"DAQmx Stop Task.vi"("task/channels in"=w799, "error in"=w797) -> ("error out"=w798:errorcluster)  [unwired: 13 out]
                }
              }
            }
          }
        }
        frame #13 {
          # "Stop 5 channel pulser CTRs"
          n307 = Unbundle By Name(w801) -> ("Dig Config"=w800:T10)
          n308 = case shown="\"Single channel\", Default" w800 {
            tunnel: w803 -> [w807 w816]
            tunnel: w804 -> [w806 _]
            tunnel: w802 -> [w805 _]
            frame "Single channel", Default {
              n309 = case shown="\"WCM Main\", Default" w806 {
                tunnel: w807 -> [w810 w813]
                tunnel: w805 -> [w809 _]
                frame "WCM Main", Default {
                  n310 = Unbundle By Name(w809) -> ("Sub Ap Excite?"=w808:bool)
                  n311 = case shown="True" w808 {
                    tunnel: w810 -> [_ w811]
                    frame False {
                    }
                    frame True {
                      n312 = for {
                        tunnel: w811 -> [w812] mode=indexing
                        n313 = call <vilib>:"DAQmx Stop Task.vi"("task/channels in"=w812) -> ()  [unwired: 13 in, 2 out]
                      }
                    }
                  }
                }
                frame "CUMC RT" {
                  n314 = for {
                    tunnel: w813 -> [w814] mode=indexing
                    n315 = call <vilib>:"DAQmx Stop Task.vi"("task/channels in"=w814) -> ()  [unwired: 13 in, 2 out]
                  }
                }
              }
            }
            frame "5-CH pulser w/ ann array" {
              n316 = case shown="False" FALSE {
                tunnel: w816 -> [_ w817]
                frame False {
                }
                frame True {
                  n317 = for {
                    tunnel: w817 -> [w818] mode=indexing
                    n318 = call <vilib>:"DAQmx Stop Task.vi"("task/channels in"=w818) -> ()  [unwired: 13 in, 2 out]
                  }
                }
              }
            }
          }
        }
        frame #14 {
          n319 = case shown="13" w825 {
            tunnel: w823 -> [_ w833 w856]
            tunnel: w824 -> [_ w848 w866]
            tunnel: w822 -> [_ w830 w849]
            tunnel: w821 -> [_ w828 _]
            tunnel: w820 -> [_ w827 _]
            tunnel: w819 -> [_ w826 _]
            frame 0, Default {
            }
            frame 13 {
              # "Save EKG data in file Ring 1 to x or solo name. Data is written as I16 binary over the first RF line. Could possible go into second line depending on how many RF pts and how many lines were acquired. Number of EKG points equals number of lines and data is acquired at PRF rate."
              n320 = call "FindLineMod.vi"("Ann Array Params"=w827, "lines per plane in"=w826, "Digitizer Settings"=w828) -> ("lines per plane mod out"=w829:i32)  [unwired: 8 in]
              n321 = call-poly <vilib>:"DAQmx Read.vi"("task/channels in"=w833, "number of samples per channel"=w829) -> ("task out"=w832:refnum<k21>, "data"=w843:i16[][], "error out"=w831:errorcluster)  [unwired: 1 in, 10 out]
              n322 = Index Array(array=w848) -> (element=w847:string)  [unwired: 1 in]
              n323 = call <vilib>:"DAQmx Stop Task.vi"("task/channels in"=w832, "error in"=w831) -> ()  [unwired: 14 out]
              n324 = Concatenate Strings(w847, ".tmp") -> (w845:string)
              n325 = Build Path(base path=w830, name or relative path=w845) -> (appended path=w844:path)
              n326 = Open/Create/Replace File(file path (use dialog)=w844) -> (refnum out=w837:refnum<file>, error out=w838:errorcluster)  [unwired: 1 in, 5 out]
              n327 = Set File Position(offset (in bytes) (0)=i64 1024, refnum=w837, error in=w838) -> (refnum out=w836:refnum<file>, error out=w835:errorcluster)  [unwired: 1 out]
              n328 = Write to Binary File(file (use dialog)=w836, data=w843, error in=w835, 5:FALSE ("prepend array or string size? (T)"), 9:T18."little-endian" ("byte order (0:big-endian, network order)")) -> (refnum out=w839:refnum<file>, error out=w840:errorcluster)  [unwired: 2 out]
              n329 = Close File(refnum=w839, error in=w840) -> ()  [unwired: 2 out]
            }
            frame 14 {
              # "Save IQ channel data from ao1 to *.IQ file. Data is written as I16 binary over the first RF line. Data saved in row format and full retrospective stage is saved in one file."
              n330 = call-poly <vilib>:"DAQmx Read.vi"("task/channels in"=w856, "timeout"=2) -> ("task out"=w854:refnum<k21>, "data"=w861:i16[][], "error out"=w850:errorcluster)  [unwired: 2 in, 9 out]
              n331 = Index Array(array=w866) -> (element=w865:string)  [unwired: 1 in]
              n332 = call <vilib>:"DAQmx Stop Task.vi"("task/channels in"=w854, "error in"=w850) -> ()  [unwired: 14 out]
              n333 = Concatenate Strings(w865, ".IQ") -> (w863:string)
              n334 = Build Path(base path=w849, name or relative path=w863) -> (appended path=w862:path)
              n335 = Open/Create/Replace File(file path (use dialog)=w862, operation (0:open)=T19."open or create") -> (refnum out=w853:refnum<file>, error out=w852:errorcluster)  [unwired: 1 in, 4 out]
              n336 = Write to Binary File(file (use dialog)=w853, data=w861, error in=w852, 5:FALSE ("prepend array or string size? (T)"), 9:T18."little-endian" ("byte order (0:big-endian, network order)")) -> (refnum out=w857:refnum<file>, error out=w858:errorcluster)  [unwired: 2 out]
              n337 = Close File(refnum=w857, error in=w858) -> ()  [unwired: 2 out]
            }
          }
        }
        frame #15 {
          n338 = case shown="True" w872 {
            tunnel: w871 -> [w873 _]
            tunnel: w870 -> [_ w879]
            tunnel: w869 -> [_ w878]
            tunnel: w868 -> [_ w877]
            tunnel: w867 -> [w874 w875]
            frame False {
              # "turn off function generator prf"
              n339 = call "PRF_Off.vi"("Location"=w873, "Motion Settings In"=w874) -> ()  [unwired: 9 in, 1 out]
            }
            frame True {
              n340 = Unbundle By Name(w875) -> ("Motion System"=w876:T5)
              n341 = case shown="\"Galil\"" w876 {
                tunnel: w879 -> [_ w880 _]
                tunnel: w877 -> [_ w882 w913]
                tunnel: w875 -> [_ w881 w911]
                frame "MM3000", "Newport ESP", "No Motion Card" {
                }
                frame "NI 735x", Default {
                  n342 = disable-structure shown="Disabled" {
                    disable-tunnel: w882 -> [w887 _]
                    disable-tunnel: w881 -> [w885 _]
                    disable-tunnel: w880 -> [w883 _]
                    frame Disabled {
                      # "Stop program"
                      n343 = Unbundle By Name(w885) -> ("Motion Bd ID"=w884:u8)
                      n344 = case shown="True" FALSE {
                        tunnel: [w896 w900] -> w889
                        tunnel: [_ w899] -> w888
                        tunnel: w884 -> [w896 w897]
                        tunnel: w887 -> [_ w898]
                        frame False {
                        }
                        frame True {
                          n345 = call-poly <vilib>:"Wait for Move Complete.flx"("Poll Interval (20 ms)"=20, "Timeout (10000 ms)"=15000, "Axis or Vector Space"=w898, "Board ID"=w897) -> ("error out"=w899:errorcluster, "Bd ID Out"=w900:T27)  [unwired: 2 in, 4 out]
                        }
                      }
                      n346 = Select(t=7, s=w883, f=6) -> (s? t:f=w894:i32)
                      n347 = call <vilib>:"Stop Program.flx"("error in (no error)"=w888, "Program (1)"=w894, "Board ID"=w889) -> ("error out"=w890:errorcluster, "Bd ID Out"=w891:T27)  [unwired: 4 out]
                      n348 = call <vilib>:"Enable Breakpoint Output.flx"("Enable Breakpoint"=FALSE, "error in (no error)"=w890, "Axis or Encoder"=w887, "Board ID"=w891) -> ()  [unwired: 6 out]
                    }
                    frame Enabled {
                    }
                  }
                }
                frame "Galil" {
                  # "Stop program"
                  n349 = Unbundle By Name(w911) -> ("GL Ref Out"=w910:refnum<k7>)
                  n350 = case shown="False" FALSE {
                    tunnel: [w914 w918] -> w904
                    tunnel: [_ w917] -> w905
                    tunnel: w910 -> [w914 w919]
                    tunnel: w913 -> [_ w916]
                    frame False {
                    }
                    frame True {
                      n351 = Decrement(x=w916) -> (x-1=w915:i32)
                      n352 = call "GL CheckForMotion.vi"("Axis"=w915, "Refnum in"=w919) -> ("error out"=w917:errorcluster, "Refnum out"=w918:refnum<k7>)  [unwired: 7 in, 1 out]
                    }
                  }
                  n353 = call "GL Command Set.vi"("Command"=Command_Menu."Halt Execute", "error in (no error)"=w905, "Value"=-1, "Galil.IGalil"=w904) -> ("error out"=w907:errorcluster, "ref out"=w908:refnum<k7>)  [unwired: 3 in, 3 out]
                  n354 = call "GL Command Set.vi"("Command"=Command_Menu."OC Off", "error in (no error)"=w907, "Galil.IGalil"=w908) -> ()  [unwired: 4 in, 5 out]
                }
              }
              n355 = case shown="1, Default" w878 {
                tunnel: w875 -> [_ w921]
                frame 0 {
                }
                frame 1, Default {
                  w922 = u16 1 items=["Function Gen Input", "Motion Trig", "Internal RT Motion Trig", "Internal CTR 1 Output"] ("Trig Source")
                  # "turn off route CT1 Trigger through 4to1 switch"
                  n356 = Unbundle By Name(w921) -> ("GL Ref Out"=w920:refnum<k7>)
                  n357 = call "RouteTrigSource.vi"("Galil.IGalil"=w920, "Trig Source"=w922) -> ()  [unwired: 9 in, 1 out]
                }
              }
            }
          }
        }
        frame #16 {
          n358 = Unbundle By Name(w924) -> ("One Way Scan"=w923:bool)
          n359 = Equal To 0?(x=w928) -> (x = 0?=w929:bool)
          n360 = case shown="\"Therapy With Scan\", Default" w926 {
            tunnel: [w932 FALSE] -> w925
            tunnel: w923 -> [w932 _]
            frame "Therapy With Scan", Default {
            }
            frame "M scan", "M Scan With Therapy Burst" {
            }
          }
          n361 = And(x=w929, y=w925) -> (x .and. y?=w927:bool)
          n362 = case shown="True" w927 {
            tunnel: w931 -> [_ w937]
            tunnel: [_ w936] -> w930
            tunnel: w924 -> [_ w935]
            frame False {
            }
            frame True {
              # "Ensure one way scanning. After forward scan, return motor to start. This ensures scanning in only one direction"
              n363 = Unbundle By Name(w935) -> ("Motion System"=w934:T5)
              n364 = case shown="\"NI 735x\", Default" w934 {
                tunnel: w937 -> [_ w939 w977 _]
                tunnel: [_ w940 FALSE ("Error Status") w994] -> w936
                tunnel: w935 -> [_ w938 w982 w993]
                frame "MM3000", "No Motion Card" {
                }
                frame "NI 735x", Default {
                  n365 = disable-structure shown="Disabled" {
                    disable-tunnel: [w957 _] -> w940
                    disable-tunnel: w939 -> [w956 _]
                    disable-tunnel: w938 -> [w943 _]
                    frame Disabled {
                      n366 = Unbundle By Name(w943) -> ("Motion Bd ID"=w942:u8, "Reverse One Way Scan"=w941:bool)
                      n367 = case shown="False" FALSE {
                        tunnel: w956 -> [_ w967]
                        tunnel: [_ w966] -> w955
                        tunnel: [w962 w965] -> w954
                        tunnel: w942 -> [w962 w963]
                        frame False {
                        }
                        frame True {
                          n368 = call <vilib>:"Load Velocity.flx"("Velocity (10000)"=10000, "Axis or Vector Space"=w967, "Board ID"=w963) -> ("error out"=w966:errorcluster, "Bd ID Out"=w965:T27)  [unwired: 4 in, 1 out]
                        }
                      }
                      n369 = Select(t=6, s=w941, f=7) -> (s? t:f=w944:i32)
                      n370 = call <vilib>:"Run Program.flx"("error in (no error)"=w955, "Program (1)"=w944, "Board ID"=w954) -> ("error out"=w961:errorcluster, "Bd ID Out"=w949:T27)  [unwired: 4 out]
                      n371 = stacked-sequence {
                        tunnel: w949 -> [w968]
                        tunnel: [w968] -> w948
                        frame #0 {
                          n372 = Wait (ms)(milliseconds to wait=u32 40) -> ()  [unwired: 1 out]
                        }
                      }
                      n373 = call-poly <vilib>:"Wait for Move Complete.flx"("Poll Interval (20 ms)"=20, "Timeout (10000 ms)"=15000, "error in (no error)"=w961, "Axis or Vector Space"=w956, "Board ID"=w948) -> ("error out"=w951:errorcluster, "Bd ID Out"=w952:T27)  [unwired: 1 in, 4 out]
                      n374 = call <vilib>:"Stop Program.flx"("error in (no error)"=w951, "Program (1)"=w944, "Board ID"=w952) -> ("error out"=w959:errorcluster, "Bd ID Out"=w960:T27)  [unwired: 4 out]
                      n375 = call <vilib>:"Read Communication Status.flx"("error in (no error)"=w959, "Board ID"=w960) -> ("error out"=w958:errorcluster)  [unwired: 6 out]
                      n376 = Unbundle By Name(w958) -> ("status"=w957:bool)
                    }
                    frame Enabled {
                    }
                  }
                }
                frame "Galil" {
                  n377 = Unbundle By Name(w982) -> ("Reverse One Way Scan"=w981:bool)
                  n378 = Unbundle By Name(w982) -> ("GL Ref Out"=w988:refnum<k7>)
                  n379 = Select(t="#FORMOD" ("Program Name"), s=w981, f="#BACKMOD" ("Program Name")) -> (s? t:f=w989:string)
                  n380 = Select(t=u8 6 ("Motion Program"), s=w981, f=u8 7 ("Motion Program")) -> (s? t:f=w972:u8)
                  n381 = call "GL Command Set.vi"("Command"=Command_Menu."Execute", "Text Input"=w989, "Value"=w972, "Galil.IGalil"=w988) -> ("error out"=w980:errorcluster, "ref out"=w978:refnum<k7>)  [unwired: 3 in, 3 out]
                  n382 = stacked-sequence {
                    tunnel: w980 -> [w990]
                    tunnel: [w990] -> w979
                    frame #0 {
                      n383 = Wait (ms)(milliseconds to wait=u32 40) -> ()  [unwired: 1 out]
                    }
                  }
                  n384 = Decrement(x=w977) -> (x-1=w976:i32)
                  n385 = call "GL CheckForMotion.vi"("error in"=w979, "Axis"=w976, "Refnum in"=w978) -> ("error out"=w973:errorcluster, "Refnum out"=w974:refnum<k7>)  [unwired: 6 in, 1 out]
                  n386 = call "GL Command Set.vi"("Command"=Command_Menu."Halt Execute", "error in (no error)"=w973, "Value"=-1, "Galil.IGalil"=w974) -> ()  [unwired: 3 in, 5 out]
                }
                frame "Newport ESP" {
                  n387 = Unbundle By Name(w993) -> ("ESP VISA"=w992:refnum<visa-resource-name>)
                  n388 = call <instrlib>:"Execute Program.vi"("Program Name"="2", "VISA resource name"=w992) -> ("error out"=w996:errorcluster, "VISA resource name out"=w998:refnum<visa-resource-name>)  [unwired: 4 in]
                  n389 = call <instrlib>:"Wait.vi"("error in (no error)"=w996, "Delay (0ms)"=20, "VISA resource name"=w998) -> ("VISA resource name out"=w995:refnum<visa-resource-name>)  [unwired: 3 in, 1 out]
                  n390 = call "WaitStopEPS.vi"("VISA resource name"=w995) -> ("Error Status"=w994:bool)  [unwired: 2 in, 2 out]
                }
              }
            }
          }
          "Motion error" <- w930
        }
        frame #17 {
          n391 = Unbundle By Name(w1003) -> ("Motion System"=w1002:T5)
          n392 = Unbundle By Name(w1000) -> ("Main Digitizer"=w1001:T9)
          n393 = case shown="\"NI 735x\"" w1002 {
            tunnel: w1005 -> [_ w1013 _]
            tunnel: w1003 -> [w1011 _ w1015]
            frame "Galil", Default {
              n394 = Unbundle By Name(w1011) -> ("GL Ref Out"=w1010:refnum<k7>)
              n395 = call "GL Command Set.vi"("Command"=Command_Menu."OC Off", "Galil.IGalil"=w1010) -> ("error out"=w1007:errorcluster, "ref out"=w1008:refnum<k7>)  [unwired: 5 in, 3 out]
              n396 = call "GL Command Set.vi"("Command"=Command_Menu."Clear Bit", "error in (no error)"=w1007, "Value"=19, "Galil.IGalil"=w1008) -> ()  [unwired: 3 in, 5 out]
            }
            frame "No Motion Card" {
              n397 = call-poly <vilib>:"DAQmx Write.vi"("task/channels in"=w1013, "data"=FALSE ("stop (T)")) -> ()  [unwired: 11 in, 3 out]
            }
            frame "NI 735x" {
              n398 = disable-structure shown="Disabled" {
                disable-tunnel: w1015 -> [w1017 _]
                frame Disabled {
                  # "Ensure breakpoints are low again"
                  n399 = Unbundle By Name(w1017) -> ("Motion Bd ID"=w1016:u8)
                  n400 = call-poly <vilib>:"Set Breakpoint Output MOMO.flx"("Must Off (False)"=T14 {"1"=TRUE, "2"=TRUE, "3"=TRUE, "4"=TRUE, "5"=TRUE, "6"=TRUE, "7"=TRUE, "8"=TRUE}, "Board ID"=w1016) -> ()  [unwired: 5 in, 3 out]
                }
                frame Enabled {
                }
              }
            }
          }
          n401 = case shown="\"AlazarTech\"" w1001 {
            tunnel: w1000 -> [_ w1021 w1024]
            tunnel: w1004 -> [_ _ w1026]
            frame "Acqiris Digitizer", Default {
            }
            frame "NI Digitizer" {
              # "Log records done after scan. Main use is for bulk indexes to account for overshoot triggers"
              n402 = Unbundle By Name(w1021) -> ("Digitizer ID Cluster.NI Instr Handles"=w1020:refnum<k15>[])
              n403 = Index Array(array=w1020) -> (element=w1019:refnum<k15>)  [unwired: 1 in]
              n404 = property class="niScope"(reference=w1019) -> ("Records Done"=w1022:i32)  [unwired: 1 in, 2 out]
              "Record Index" <- w1022
              n405 = Decrement(x=w1022) -> ()  [unwired: 1 out]
            }
            frame "AlazarTech" {
              n406 = Unbundle By Name(w1024) -> ("Digitizer ID Cluster.Acqiris/Alazar/SP ID"=w1023:u32[])
              n407 = Unbundle By Name(w1026) -> ("data value reference"=w1025:refnum<data-value>)
              n408 = Delete Data Value Reference(data value reference=w1025) -> ()  [unwired: 1 in, 2 out]
              n409 = for {
                tunnel: w1023 -> [w1027] mode=indexing
                n410 = call "AlazarAbortAsyncRead.vi"("Handle"=w1027) -> ()  [unwired: 1 in, 3 out]
              }
            }
          }
        }
      }
      "Timeout" <- w45
    }
    frame True {
    }
  }
